vi "tdo -- V2.vi"() -> ()   [LabVIEW 2021]
uses:
  3-lorentzian-parameters.ctl
  filename-action.ctl
  nameformattingitem.ctl
  agregator -- action.ctl
  interpolation state - real.ctl
  tdo -- new/Data window.ctl
  <vilib>/Analysis/4window.llb/Hanning Window (DBL).vi
  <vilib>/Analysis/4window.llb/Blackman Window (DBL).vi
  linear interpolation - real -- V2.vi
  <vilib>/Analysis/4window.llb/AllCosWindow (DBL).vi
  <vilib>/Analysis/baseanly.llb/A x B.vi
  <vilib>/Analysis/baseanly.llb/Real A x B.vi
  Q -- check range -- i -- real.vi
  line -- complex.vi
  Q -- check range -- i -- integer.vi
  Q - not nan -- real.vi
  Q - not nan -- integer.vi
  <vilib>/measure/matone.llb/Extract Single Tone Information 1 Chan.vi
  <vilib>/Waveform/WDTOps.llb/WDT Number of Waveform Samples DBL.vi
  <vilib>/Utility/file.llb/Write Delimited Spreadsheet (string).vi
  <vilib>/Analysis/Matrix/Numeric/Conversions/Array To Matrix.vi
  <vilib>/Analysis/Matrix/Numeric/Conversions/Array To Matrix - RA2.vi
  <vilib>/Analysis/baseanly.llb/Inverse Matrix.vi
  <vilib>/Analysis/baseanly.llb/Real Inverse Matrix.vi
  <vilib>/Utility/file.llb/Write Delimited Spreadsheet (DBL).vi
  <vilib>/Analysis/NI_AALPro.lvlib
  <vilib>/measure/NI_MAPro.lvlib
  <vilib>/Analysis/NI_AAL_SigProc.lvlib
panel:
  in  "Tab Control":enum32{"Page 1", "Page 2", "Page 3", "Page 4"}(tab)
  in  "Tab Control 2":enum32{"Page 1", "Page 2"}(tab)
  in  "file pattern":string="p_c3*.tdms"
  in  "main folder":path=path "/Users/arkadyshekhter/Library/CloudStorage/Dropbox/shared_KimValBra/UTe2--Apr2024/april_2024"
  in  "readmathstring":bool=TRUE
  in  "selection :|\\":u16(ring)=31 caption="files" items=["p_c3_008_040924.tdms", "p_c3_003_041124.tdms", "p_c3_004_042224.tdms", "p_c3_005_042224.tdms", "p_c3_006_042224.tdms", "p_c3_007_042224.tdms", "p_c3_010_040924.tdms", "p_c3_008_042224.tdms", "p_c3_013_041024.tdms", "p_c3_004_041124.tdms", "p_c3_009_042224.tdms", "p_c3_006_041124.tdms", "p_c3_011_040924.tdms", "p_c3_010_042224.tdms", "p_c3_005_041124.tdms", "p_c3_012_041024.tdms", "p_c3_011_041024.tdms", "p_c3_002_041024.tdms", "p_c3_010_041024.tdms", "p_c3_009_041024.tdms", "p_c3_008_042524.tdms", "p_c3_007_041124.tdms", "p_c3_003_041024.tdms", "p_c3_007_042524.tdms", "p_c3_008_041124.tdms", "p_c3_006_042524.tdms", "p_c3_008_041024.tdms", "p_c3_005_042524.tdms", "p_c3_004_042524.tdms", "p_c3_007_041024.tdms", "p_c3_010_041124.tdms", "p_c3_003_041224.tdms", "p_c3_004_041224.tdms", "p_c3_005_041224.tdms", "p_c3_006_041224.tdms", "p_c3_007_041224.tdms", "p_c3_008_041224.tdms", "p_c3_009_041224.tdms", "p_c3_009_041124.tdms", "p_c3_011_041124.tdms", "p_c3_003_042524.tdms", "p_c3_004_041024.tdms", "p_c3_011_042224.tdms", "p_c3_013_042224.tdms", "p_c3_006_041024.tdms", "p_c3_002_041224.tdms", "p_c3_002_042524.tdms", "p_c3_004_042424.tdms", "p_c3_005_041024.tdms"]
  in  "file":path=path "/Users/arkadyshekhter/Library/CloudStorage/Dropbox/shared_KimValBra/UTe2--Apr2024/041224/p_c3_008_041224.tdms"
  out "T (K)":dbl=15.0 format="%#_3f"
  out "B (T)":dbl=60.0 format="%#_3f"
  out "θ (deg)":dbl=153.0 format="%#_3f"
  out "key":string="008_041224"
  in  "dothething! :' '":bool=TRUE
  in  "gamma window (sec)":dbl(slide)=0.00043000000000000004 scale=5e-05..0.001 scale format="%#_3p"
  out "E":cluster{dbl[], dbl[]}(graph)
  out "C":cluster{dbl[], dbl[]}(graph)
  out "A":cluster{dbl[], dbl[]}(graph)
  out "B":waveform(dbl)(graph)={"t0"=timestamp(-0.00999989999999995 s since 1904-01-01), "dt"=2e-05, "Y"=[]}
  out "Progress":dbl(slide)=1.004382311063316 scale=0.0..1.0
  in  "?":T1(tab)=enum."selectros"
  in  "Power spctr. threshold":dbl=0.0001 format="%.2p"
  in  "Freq. threshold":dbl=30000.0 format="%#_3p"
  in  "window width (s)":dbl=0.0003 format="%#_6p"
  in  "window step (s)":dbl=2e-05 format="%#_6p"
  in  "detection method":T2(ring)
  in  "fit width":i32=9 min=3
  in  "window type":enum16{"Hanning", "Box", "Blackman"}(ring)
  in  "what?":T3={"ignore set of !"=TRUE, "set (1T|2B)"=0, "ignore θ !"=TRUE, "ignore B !"=TRUE, "T (K)"=1.0, "ignore T !"=TRUE, "θ (∘)"=0.0, "B (T)"=0.0, "lookup"={"set of lookup"={0=1.0, 1=2.0}, "all set of"={0.0}, "T lookup"={0=0.12, 1=0.122, 2=0.14, 3=0.148, 4=0.15, 5=0.157, 6=0.16, 7=0.168, 8=0.17, 9=0.178, 10=0.179, 11=0.18, 12=0.19, 13=0.197, 14=0.2, 15=0.249, 16=0.25, 17=0.255, 18=0.26, 19=0.3, 20=0.307, 21=0.308, 22=0.31, 23=0.36, 24=0.42, 25=0.43, 26=0.438, 27=0.512, 28=0.52, 29=0.53, 30=0.61, 31=0.62, 32=0.63, 33=0.677, 34=0.81, 35=0.82, 36=0.83, 37=1.0, 38=1.1, 39=1.12, 40=1.13, 41=1.25, 42=1.28, 43=1.31, 44=1.39, 45=1.5, 46=1.52, 47=1.55, 48=1.6, 49=1.7, 50=1.8, 51=1.9, 52=2.1, 53=2.3, 54=3.0, 55=3.07, 56=3.1, 57=3.11, 58=5.5, 59=5.7, 60=5.75}, "θ lookup"={0=0.0, 1=30.0, 2=45.0, 3=60.0, 4=90.0}, "B lookup"={0=0.0, 1=1.0, 2=2.0, 3=4.0, 4=5.0, 5=6.0, 6=7.0, 7=8.0, 8=9.0, 9=10.0, 10=11.0, 11=12.0}, "all T's"={4.0, 10.0, 15.0, 17.0, 20.0, 25.0, 30.0}, "all θ's"={0.0, 15.0, 20.0, 25.0, 30.0, 40.0, 45.0, 50.0, 53.0, 55.0, 60.0, 65.0, 67.0, 75.0, 85.0, 90.0, 95.0, 105.0, 112.0, 120.0, 128.0, 135.0, 150.0, 151.0, 153.0, 155.0, 157.0, 160.0, 163.0, 165.0, 170.0, 180.0}, "all B's"={60.0}, "all sides"={4000.0, 8000.0}, "side lookup"={0=4000.0, 1=8000.0}}} {"B (T)" items=["0.000", "1.000", "2.000", "4.000", "5.000", "6.000", "7.000", "8.000", "9.000", "10.000", "11.000", "12.000"]; "θ (∘)" items=["0.000", "30.000", "45.000", "60.000", "90.000"]; "T (K)" items=["0.120", "0.122", "0.140", "0.148", "0.150", "0.157", "0.160", "0.168", "0.170", "0.178", "0.179", "0.180", "0.190", "0.197", "0.200", "0.249", "0.250", "0.255", "0.260", "0.300", "0.307", "0.308", "0.310", "0.360", "0.420", "0.430", "0.438", "0.512", "0.520", "0.530", "0.610", "0.620", "0.630", "0.677", "0.810", "0.820", "0.830", "1.000", "1.100", "1.120", "1.130", "1.250", "1.280", "1.310", "1.390", "1.500", "1.520", "1.550", "1.600", "1.700", "1.800", "1.900", "2.100", "2.300", "3.000", "3.070", "3.100", "3.110", "5.500", "5.700", "5.750"]; "set (1T|2B)" items=["1", "2"]}
  in  "X selector":T4=enum."θ (deg)"
  in  "ovewrite file?":bool=TRUE
  in  "add file suffix":string="_tdo_"
  in  "remove file prefix":string="p_c3_"
  out "first line":string[](array[string])=["<Not A Path>_time <Not A Path>_field <Not A Path>_freq <Not A Path>_amp <Not A Path>_gamma "]
  in  "field channel name":string="Field"
  in  "group name":string="p"
  in  "signal channel name":string="Vpick"
  in  "Field correction":dbl=1.0
  in  "Length for Bdot offset, s":dbl=0.009 format="%#_6p"
  out "D":waveform(dbl)(graph)={"t0"=timestamp(-0.00999989999999995 s since 1904-01-01), "dt"=2e-05, "Y"=[]}
  in  "Exit!":bool=TRUE
  in  "Low-pass filter":T5={"Clip IIR filter ramps, in 1/Tc units"=1.0, "Two-pass & flip"=TRUE, "IIR filter specifications"={"Topology"=enum."Off", "Type"=enum."Lowpass", "Order"=1, "Lower Fc"=1e-06, "Upper Fc"=0.0, "PB Ripple"=1.0, "SB Attenuation"=60.0}} {"IIR filter specifications"."PB Ripple" format="%0.2f"; "IIR filter specifications"."Lower Fc" format="%0.2p"; "IIR filter specifications"."SB Attenuation" format="%0.2f"; "IIR filter specifications"."Upper Fc" format="%0.2p"}
  in  "# of threads":i32=4
  out "Field profile":waveform(dbl)(graph)={"t0"=timestamp(-0.00999989999999995 s since 1904-01-01), "dt"=2e-05, "Y"=[]}
  out "all short filenames":map{string, string}(c390)={"002_041024"="p_c3_002_041024.tdms", "002_041224"="p_c3_002_041224.tdms", "002_042424"="p_c3_002_042424.tdms", "003_041024"="p_c3_003_041024.tdms", "003_041124"="p_c3_003_041124.tdms", "003_041224"="p_c3_003_041224.tdms", "003_042424"="p_c3_003_042424.tdms", "004_041024"="p_c3_004_041024.tdms", "004_041124"="p_c3_004_041124.tdms", "004_041224"="p_c3_004_041224.tdms", "004_042224"="p_c3_004_042224.tdms", "004_042424"="p_c3_004_042424.tdms", "005_041024"="p_c3_005_041024.tdms", "005_041124"="p_c3_005_041124.tdms", "005_041224"="p_c3_005_041224.tdms", "005_042224"="p_c3_005_042224.tdms", "006_041024"="p_c3_006_041024.tdms", "006_041124"="p_c3_006_041124.tdms", "006_041224"="p_c3_006_041224.tdms", "006_042224"="p_c3_006_042224.tdms", "007_041024"="p_c3_007_041024.tdms", "007_041124"="p_c3_007_041124.tdms", "007_041224"="p_c3_007_041224.tdms", "007_042224"="p_c3_007_042224.tdms", "008_040924"="p_c3_008_040924.tdms", "008_041024"="p_c3_008_041024.tdms", "008_041124"="p_c3_008_041124.tdms", "008_041224"="p_c3_008_041224.tdms", "008_042224"="p_c3_008_042224.tdms", "009_041024"="p_c3_009_041024.tdms", "009_041124"="p_c3_009_041124.tdms", "009_041224"="p_c3_009_041224.tdms", "009_042224"="p_c3_009_042224.tdms", "010_040924"="p_c3_010_040924.tdms", "010_041024"="p_c3_010_041024.tdms", "010_041124"="p_c3_010_041124.tdms", "010_042224"="p_c3_010_042224.tdms", "011_040924"="p_c3_011_040924.tdms", "011_041024"="p_c3_011_041024.tdms", "011_041124"="p_c3_011_041124.tdms", "011_042224"="p_c3_011_042224.tdms", "012_041024"="p_c3_012_041024.tdms", "013_041024"="p_c3_013_041024.tdms", "013_042224"="p_c3_013_042224.tdms"}
  out "temps&degs":map{string, map{T4, dbl}}(c390)={"002_041024"={enum."T (K)"=4.0, enum."B (T)"=60.0, enum."θ (deg)"=90.0, enum."plain"=23.0, enum."vproj"=0.0}, "002_041224"={enum."T (K)"=4.0, enum."B (T)"=60.0, enum."θ (deg)"=170.0, enum."plain"=23.0, enum."vproj"=-0.69}, "002_042424"={enum."T (K)"=4.0, enum."B (T)"=60.0, enum."θ (deg)"=170.0, enum."plain"=13.0, enum."vproj"=-0.692}, "003_041024"={enum."T (K)"=4.0, enum."B (T)"=60.0, enum."θ (deg)"=120.0, enum."plain"=23.0, enum."vproj"=-0.34}, "003_041124"={enum."T (K)"=4.0, enum."B (T)"=60.0, enum."θ (deg)"=15.0, enum."plain"=23.0, enum."vproj"=0.673}, "003_041224"={enum."T (K)"=4.0, enum."B (T)"=60.0, enum."θ (deg)"=153.0, enum."plain"=23.0, enum."vproj"=-0.625}, "003_042424"={enum."T (K)"=4.0, enum."B (T)"=60.0, enum."θ (deg)"=160.0, enum."plain"=13.0, enum."vproj"=-0.662}, "004_041024"={enum."T (K)"=4.0, enum."B (T)"=60.0, enum."θ (deg)"=160.0, enum."plain"=23.0, enum."vproj"=-0.663}, "004_041124"={enum."T (K)"=4.0, enum."B (T)"=60.0, enum."θ (deg)"=50.0, enum."plain"=23.0, enum."vproj"=0.442}, "004_041224"={enum."T (K)"=10.0, enum."B (T)"=60.0, enum."θ (deg)"=153.0, enum."plain"=23.0, enum."vproj"=-0.625}, "004_042224"={enum."T (K)"=4.0, enum."B (T)"=60.0, enum."θ (deg)"=15.0, enum."plain"=23.0, enum."vproj"=0.67}, "004_042424"={enum."T (K)"=4.0, enum."B (T)"=60.0, enum."θ (deg)"=180.0, enum."plain"=13.0, enum."vproj"=-0.702}, "005_041024"={enum."T (K)"=4.0, enum."B (T)"=60.0, enum."θ (deg)"=180.0, enum."plain"=23.0, enum."vproj"=-0.699}, "005_041124"={enum."T (K)"=4.0, enum."B (T)"=60.0, enum."θ (deg)"=67.0, enum."plain"=23.0, enum."vproj"=0.269}, "005_041224"={enum."T (K)"=20.0, enum."B (T)"=60.0, enum."θ (deg)"=153.0, enum."plain"=23.0, enum."vproj"=-0.625}, "005_042224"={enum."T (K)"=4.0, enum."B (T)"=60.0, enum."θ (deg)"=20.0, enum."plain"=23.0, enum."vproj"=0.651}, "006_041024"={enum."T (K)"=4.0, enum."B (T)"=60.0, enum."θ (deg)"=165.0, enum."plain"=23.0, enum."vproj"=-0.677}, "006_041124"={enum."T (K)"=4.0, enum."B (T)"=60.0, enum."θ (deg)"=55.0, enum."plain"=23.0, enum."vproj"=0.397}, "006_041224"={enum."T (K)"=30.0, enum."B (T)"=60.0, enum."θ (deg)"=153.0, enum."plain"=23.0, enum."vproj"=-0.625}, "006_042224"={enum."T (K)"=4.0, enum."B (T)"=60.0, enum."θ (deg)"=25.0, enum."plain"=23.0, enum."vproj"=0.628}, "007_041024"={enum."T (K)"=4.0, enum."B (T)"=60.0, enum."θ (deg)"=150.0, enum."plain"=23.0, enum."vproj"=-0.603}, "007_041124"={enum."T (K)"=4.0, enum."B (T)"=60.0, enum."θ (deg)"=112.0, enum."plain"=23.0, enum."vproj"=-0.26}, "007_041224"={enum."T (K)"=25.0, enum."B (T)"=60.0, enum."θ (deg)"=153.0, enum."plain"=23.0, enum."vproj"=-0.625}, "007_042224"={enum."T (K)"=4.0, enum."B (T)"=60.0, enum."θ (deg)"=30.0, enum."plain"=23.0, enum."vproj"=0.603}, "008_040924"={enum."T (K)"=4.0, enum."B (T)"=60.0, enum."θ (deg)"=0.0, enum."plain"=23.0, enum."vproj"=0.69}, "008_041024"={enum."T (K)"=4.0, enum."B (T)"=60.0, enum."θ (deg)"=135.0, enum."plain"=23.0, enum."vproj"=-0.496}, "008_041124"={enum."T (K)"=4.0, enum."B (T)"=60.0, enum."θ (deg)"=128.0, enum."plain"=23.0, enum."vproj"=-0.432}, "008_041224"={enum."T (K)"=15.0, enum."B (T)"=60.0, enum."θ (deg)"=153.0, enum."plain"=23.0, enum."vproj"=-0.625}, "008_042224"={enum."T (K)"=4.0, enum."B (T)"=60.0, enum."θ (deg)"=40.0, enum."plain"=23.0, enum."vproj"=0.533}, "009_041024"={enum."T (K)"=4.0, enum."B (T)"=60.0, enum."θ (deg)"=105.0, enum."plain"=23.0, enum."vproj"=-0.178}, "009_041124"={enum."T (K)"=4.0, enum."B (T)"=60.0, enum."θ (deg)"=155.0, enum."plain"=23.0, enum."vproj"=-0.634}, "009_041224"={enum."T (K)"=17.0, enum."B (T)"=60.0, enum."θ (deg)"=153.0, enum."plain"=23.0, enum."vproj"=-0.625}, "009_042224"={enum."T (K)"=4.0, enum."B (T)"=60.0, enum."θ (deg)"=53.0, enum."plain"=23.0, enum."vproj"=0.415}, "010_040924"={enum."T (K)"=4.0, enum."B (T)"=60.0, enum."θ (deg)"=30.0, enum."plain"=23.0, enum."vproj"=0.6}, "010_041024"={enum."T (K)"=4.0, enum."B (T)"=60.0, enum."θ (deg)"=95.0, enum."plain"=23.0, enum."vproj"=-0.057}, "010_041124"={enum."T (K)"=4.0, enum."B (T)"=60.0, enum."θ (deg)"=151.0, enum."plain"=23.0, enum."vproj"=-0.615}, "010_042224"={enum."T (K)"=4.0, enum."B (T)"=60.0, enum."θ (deg)"=65.0, enum."plain"=23.0, enum."vproj"=0.288}, "011_040924"={enum."T (K)"=4.0, enum."B (T)"=60.0, enum."θ (deg)"=60.0, enum."plain"=23.0, enum."vproj"=0.348}, "011_041024"={enum."T (K)"=4.0, enum."B (T)"=60.0, enum."θ (deg)"=85.0, enum."plain"=23.0, enum."vproj"=0.065}, "011_041124"={enum."T (K)"=4.0, enum."B (T)"=60.0, enum."θ (deg)"=157.0, enum."plain"=23.0, enum."vproj"=-0.648}, "011_042224"={enum."T (K)"=4.0, enum."B (T)"=60.0, enum."θ (deg)"=160.0, enum."plain"=23.0, enum."vproj"=-0.661}, "012_041024"={enum."T (K)"=4.0, enum."B (T)"=60.0, enum."θ (deg)"=75.0, enum."plain"=23.0, enum."vproj"=0.183}, "013_041024"={enum."T (K)"=4.0, enum."B (T)"=60.0, enum."θ (deg)"=45.0, enum."plain"=23.0, enum."vproj"=0.494}, "013_042224"={enum."T (K)"=4.0, enum."B (T)"=60.0, enum."θ (deg)"=163.0, enum."plain"=23.0, enum."vproj"=-0.674}}
  out "mathematica thing":map{string, map{T4, dbl}}(c390)={"002_041024"={enum."T (K)"=4.0, enum."B (T)"=60.0, enum."θ (deg)"=90.0, enum."plain"=23.0, enum."vproj"=0.0}, "002_041224"={enum."T (K)"=4.0, enum."B (T)"=60.0, enum."θ (deg)"=170.0, enum."plain"=23.0, enum."vproj"=-0.69}, "002_042424"={enum."T (K)"=4.0, enum."B (T)"=60.0, enum."θ (deg)"=170.0, enum."plain"=13.0, enum."vproj"=-0.692}, "003_041024"={enum."T (K)"=4.0, enum."B (T)"=60.0, enum."θ (deg)"=120.0, enum."plain"=23.0, enum."vproj"=-0.34}, "003_041124"={enum."T (K)"=4.0, enum."B (T)"=60.0, enum."θ (deg)"=15.0, enum."plain"=23.0, enum."vproj"=0.673}, "003_041224"={enum."T (K)"=4.0, enum."B (T)"=60.0, enum."θ (deg)"=153.0, enum."plain"=23.0, enum."vproj"=-0.625}, "003_042424"={enum."T (K)"=4.0, enum."B (T)"=60.0, enum."θ (deg)"=160.0, enum."plain"=13.0, enum."vproj"=-0.662}, "004_041024"={enum."T (K)"=4.0, enum."B (T)"=60.0, enum."θ (deg)"=160.0, enum."plain"=23.0, enum."vproj"=-0.663}, "004_041124"={enum."T (K)"=4.0, enum."B (T)"=60.0, enum."θ (deg)"=50.0, enum."plain"=23.0, enum."vproj"=0.442}, "004_041224"={enum."T (K)"=10.0, enum."B (T)"=60.0, enum."θ (deg)"=153.0, enum."plain"=23.0, enum."vproj"=-0.625}, "004_042224"={enum."T (K)"=4.0, enum."B (T)"=60.0, enum."θ (deg)"=15.0, enum."plain"=23.0, enum."vproj"=0.67}, "004_042424"={enum."T (K)"=4.0, enum."B (T)"=60.0, enum."θ (deg)"=180.0, enum."plain"=13.0, enum."vproj"=-0.702}, "005_041024"={enum."T (K)"=4.0, enum."B (T)"=60.0, enum."θ (deg)"=180.0, enum."plain"=23.0, enum."vproj"=-0.699}, "005_041124"={enum."T (K)"=4.0, enum."B (T)"=60.0, enum."θ (deg)"=67.0, enum."plain"=23.0, enum."vproj"=0.269}, "005_041224"={enum."T (K)"=20.0, enum."B (T)"=60.0, enum."θ (deg)"=153.0, enum."plain"=23.0, enum."vproj"=-0.625}, "005_042224"={enum."T (K)"=4.0, enum."B (T)"=60.0, enum."θ (deg)"=20.0, enum."plain"=23.0, enum."vproj"=0.651}, "006_041024"={enum."T (K)"=4.0, enum."B (T)"=60.0, enum."θ (deg)"=165.0, enum."plain"=23.0, enum."vproj"=-0.677}, "006_041124"={enum."T (K)"=4.0, enum."B (T)"=60.0, enum."θ (deg)"=55.0, enum."plain"=23.0, enum."vproj"=0.397}, "006_041224"={enum."T (K)"=30.0, enum."B (T)"=60.0, enum."θ (deg)"=153.0, enum."plain"=23.0, enum."vproj"=-0.625}, "006_042224"={enum."T (K)"=4.0, enum."B (T)"=60.0, enum."θ (deg)"=25.0, enum."plain"=23.0, enum."vproj"=0.628}, "007_041024"={enum."T (K)"=4.0, enum."B (T)"=60.0, enum."θ (deg)"=150.0, enum."plain"=23.0, enum."vproj"=-0.603}, "007_041124"={enum."T (K)"=4.0, enum."B (T)"=60.0, enum."θ (deg)"=112.0, enum."plain"=23.0, enum."vproj"=-0.26}, "007_041224"={enum."T (K)"=25.0, enum."B (T)"=60.0, enum."θ (deg)"=153.0, enum."plain"=23.0, enum."vproj"=-0.625}, "007_042224"={enum."T (K)"=4.0, enum."B (T)"=60.0, enum."θ (deg)"=30.0, enum."plain"=23.0, enum."vproj"=0.603}, "008_040924"={enum."T (K)"=4.0, enum."B (T)"=60.0, enum."θ (deg)"=0.0, enum."plain"=23.0, enum."vproj"=0.69}, "008_041024"={enum."T (K)"=4.0, enum."B (T)"=60.0, enum."θ (deg)"=135.0, enum."plain"=23.0, enum."vproj"=-0.496}, "008_041124"={enum."T (K)"=4.0, enum."B (T)"=60.0, enum."θ (deg)"=128.0, enum."plain"=23.0, enum."vproj"=-0.432}, "008_041224"={enum."T (K)"=15.0, enum."B (T)"=60.0, enum."θ (deg)"=153.0, enum."plain"=23.0, enum."vproj"=-0.625}, "008_042224"={enum."T (K)"=4.0, enum."B (T)"=60.0, enum."θ (deg)"=40.0, enum."plain"=23.0, enum."vproj"=0.533}, "009_041024"={enum."T (K)"=4.0, enum."B (T)"=60.0, enum."θ (deg)"=105.0, enum."plain"=23.0, enum."vproj"=-0.178}, "009_041124"={enum."T (K)"=4.0, enum."B (T)"=60.0, enum."θ (deg)"=155.0, enum."plain"=23.0, enum."vproj"=-0.634}, "009_041224"={enum."T (K)"=17.0, enum."B (T)"=60.0, enum."θ (deg)"=153.0, enum."plain"=23.0, enum."vproj"=-0.625}, "009_042224"={enum."T (K)"=4.0, enum."B (T)"=60.0, enum."θ (deg)"=53.0, enum."plain"=23.0, enum."vproj"=0.415}, "010_040924"={enum."T (K)"=4.0, enum."B (T)"=60.0, enum."θ (deg)"=30.0, enum."plain"=23.0, enum."vproj"=0.6}, "010_041024"={enum."T (K)"=4.0, enum."B (T)"=60.0, enum."θ (deg)"=95.0, enum."plain"=23.0, enum."vproj"=-0.057}, "010_041124"={enum."T (K)"=4.0, enum."B (T)"=60.0, enum."θ (deg)"=151.0, enum."plain"=23.0, enum."vproj"=-0.615}, "010_042224"={enum."T (K)"=4.0, enum."B (T)"=60.0, enum."θ (deg)"=65.0, enum."plain"=23.0, enum."vproj"=0.288}, "011_040924"={enum."T (K)"=4.0, enum."B (T)"=60.0, enum."θ (deg)"=60.0, enum."plain"=23.0, enum."vproj"=0.348}, "011_041024"={enum."T (K)"=4.0, enum."B (T)"=60.0, enum."θ (deg)"=85.0, enum."plain"=23.0, enum."vproj"=0.065}, "011_041124"={enum."T (K)"=4.0, enum."B (T)"=60.0, enum."θ (deg)"=157.0, enum."plain"=23.0, enum."vproj"=-0.648}, "011_042224"={enum."T (K)"=4.0, enum."B (T)"=60.0, enum."θ (deg)"=160.0, enum."plain"=23.0, enum."vproj"=-0.661}, "012_041024"={enum."T (K)"=4.0, enum."B (T)"=60.0, enum."θ (deg)"=75.0, enum."plain"=23.0, enum."vproj"=0.183}, "013_041024"={enum."T (K)"=4.0, enum."B (T)"=60.0, enum."θ (deg)"=45.0, enum."plain"=23.0, enum."vproj"=0.494}, "013_042224"={enum."T (K)"=4.0, enum."B (T)"=60.0, enum."θ (deg)"=163.0, enum."plain"=23.0, enum."vproj"=-0.674}}
  out "all full filenames":map{string, path}(c390)={"002_041024"=path "/Users/arkadyshekhter/Library/CloudStorage/Dropbox/shared_KimValBra/UTe2--Apr2024/041024/p_c3_002_041024.tdms", "002_041224"=path "/Users/arkadyshekhter/Library/CloudStorage/Dropbox/shared_KimValBra/UTe2--Apr2024/041224/p_c3_002_041224.tdms", "002_042424"=path "/Users/arkadyshekhter/Library/CloudStorage/Dropbox/shared_KimValBra/UTe2--Apr2024/042424/p_c3_002_042424.tdms", "003_041024"=path "/Users/arkadyshekhter/Library/CloudStorage/Dropbox/shared_KimValBra/UTe2--Apr2024/041024/p_c3_003_041024.tdms", "003_041124"=path "/Users/arkadyshekhter/Library/CloudStorage/Dropbox/shared_KimValBra/UTe2--Apr2024/041124/p_c3_003_041124.tdms", "003_041224"=path "/Users/arkadyshekhter/Library/CloudStorage/Dropbox/shared_KimValBra/UTe2--Apr2024/041224/p_c3_003_041224.tdms", "003_042424"=path "/Users/arkadyshekhter/Library/CloudStorage/Dropbox/shared_KimValBra/UTe2--Apr2024/042424/p_c3_003_042424.tdms", "004_041024"=path "/Users/arkadyshekhter/Library/CloudStorage/Dropbox/shared_KimValBra/UTe2--Apr2024/041024/p_c3_004_041024.tdms", "004_041124"=path "/Users/arkadyshekhter/Library/CloudStorage/Dropbox/shared_KimValBra/UTe2--Apr2024/041124/p_c3_004_041124.tdms", "004_041224"=path "/Users/arkadyshekhter/Library/CloudStorage/Dropbox/shared_KimValBra/UTe2--Apr2024/041224/p_c3_004_041224.tdms", "004_042224"=path "/Users/arkadyshekhter/Library/CloudStorage/Dropbox/shared_KimValBra/UTe2--Apr2024/042224/p_c3_004_042224.tdms", "004_042424"=path "/Users/arkadyshekhter/Library/CloudStorage/Dropbox/shared_KimValBra/UTe2--Apr2024/042424/p_c3_004_042424.tdms", "005_041024"=path "/Users/arkadyshekhter/Library/CloudStorage/Dropbox/shared_KimValBra/UTe2--Apr2024/041024/p_c3_005_041024.tdms", "005_041124"=path "/Users/arkadyshekhter/Library/CloudStorage/Dropbox/shared_KimValBra/UTe2--Apr2024/041124/p_c3_005_041124.tdms", "005_041224"=path "/Users/arkadyshekhter/Library/CloudStorage/Dropbox/shared_KimValBra/UTe2--Apr2024/041224/p_c3_005_041224.tdms", "005_042224"=path "/Users/arkadyshekhter/Library/CloudStorage/Dropbox/shared_KimValBra/UTe2--Apr2024/042224/p_c3_005_042224.tdms", "006_041024"=path "/Users/arkadyshekhter/Library/CloudStorage/Dropbox/shared_KimValBra/UTe2--Apr2024/041024/p_c3_006_041024.tdms", "006_041124"=path "/Users/arkadyshekhter/Library/CloudStorage/Dropbox/shared_KimValBra/UTe2--Apr2024/041124/p_c3_006_041124.tdms", "006_041224"=path "/Users/arkadyshekhter/Library/CloudStorage/Dropbox/shared_KimValBra/UTe2--Apr2024/041224/p_c3_006_041224.tdms", "006_042224"=path "/Users/arkadyshekhter/Library/CloudStorage/Dropbox/shared_KimValBra/UTe2--Apr2024/042224/p_c3_006_042224.tdms", "007_041024"=path "/Users/arkadyshekhter/Library/CloudStorage/Dropbox/shared_KimValBra/UTe2--Apr2024/041024/p_c3_007_041024.tdms", "007_041124"=path "/Users/arkadyshekhter/Library/CloudStorage/Dropbox/shared_KimValBra/UTe2--Apr2024/041124/p_c3_007_041124.tdms", "007_041224"=path "/Users/arkadyshekhter/Library/CloudStorage/Dropbox/shared_KimValBra/UTe2--Apr2024/041224/p_c3_007_041224.tdms", "007_042224"=path "/Users/arkadyshekhter/Library/CloudStorage/Dropbox/shared_KimValBra/UTe2--Apr2024/042224/p_c3_007_042224.tdms", "008_040924"=path "/Users/arkadyshekhter/Library/CloudStorage/Dropbox/shared_KimValBra/UTe2--Apr2024/040924/p_c3_008_040924.tdms", "008_041024"=path "/Users/arkadyshekhter/Library/CloudStorage/Dropbox/shared_KimValBra/UTe2--Apr2024/041024/p_c3_008_041024.tdms", "008_041124"=path "/Users/arkadyshekhter/Library/CloudStorage/Dropbox/shared_KimValBra/UTe2--Apr2024/041124/p_c3_008_041124.tdms", "008_041224"=path "/Users/arkadyshekhter/Library/CloudStorage/Dropbox/shared_KimValBra/UTe2--Apr2024/041224/p_c3_008_041224.tdms", "008_042224"=path "/Users/arkadyshekhter/Library/CloudStorage/Dropbox/shared_KimValBra/UTe2--Apr2024/042224/p_c3_008_042224.tdms", "009_041024"=path "/Users/arkadyshekhter/Library/CloudStorage/Dropbox/shared_KimValBra/UTe2--Apr2024/041024/p_c3_009_041024.tdms", "009_041124"=path "/Users/arkadyshekhter/Library/CloudStorage/Dropbox/shared_KimValBra/UTe2--Apr2024/041124/p_c3_009_041124.tdms", "009_041224"=path "/Users/arkadyshekhter/Library/CloudStorage/Dropbox/shared_KimValBra/UTe2--Apr2024/041224/p_c3_009_041224.tdms", "009_042224"=path "/Users/arkadyshekhter/Library/CloudStorage/Dropbox/shared_KimValBra/UTe2--Apr2024/042224/p_c3_009_042224.tdms", "010_040924"=path "/Users/arkadyshekhter/Library/CloudStorage/Dropbox/shared_KimValBra/UTe2--Apr2024/040924/p_c3_010_040924.tdms", "010_041024"=path "/Users/arkadyshekhter/Library/CloudStorage/Dropbox/shared_KimValBra/UTe2--Apr2024/041024/p_c3_010_041024.tdms", "010_041124"=path "/Users/arkadyshekhter/Library/CloudStorage/Dropbox/shared_KimValBra/UTe2--Apr2024/041124/p_c3_010_041124.tdms", "010_042224"=path "/Users/arkadyshekhter/Library/CloudStorage/Dropbox/shared_KimValBra/UTe2--Apr2024/042224/p_c3_010_042224.tdms", "011_040924"=path "/Users/arkadyshekhter/Library/CloudStorage/Dropbox/shared_KimValBra/UTe2--Apr2024/040924/p_c3_011_040924.tdms", "011_041024"=path "/Users/arkadyshekhter/Library/CloudStorage/Dropbox/shared_KimValBra/UTe2--Apr2024/041024/p_c3_011_041024.tdms", "011_041124"=path "/Users/arkadyshekhter/Library/CloudStorage/Dropbox/shared_KimValBra/UTe2--Apr2024/041124/p_c3_011_041124.tdms", "011_042224"=path "/Users/arkadyshekhter/Library/CloudStorage/Dropbox/shared_KimValBra/UTe2--Apr2024/042224/p_c3_011_042224.tdms", "012_041024"=path "/Users/arkadyshekhter/Library/CloudStorage/Dropbox/shared_KimValBra/UTe2--Apr2024/041024/p_c3_012_041024.tdms", "013_041024"=path "/Users/arkadyshekhter/Library/CloudStorage/Dropbox/shared_KimValBra/UTe2--Apr2024/041024/p_c3_013_041024.tdms", "013_042224"=path "/Users/arkadyshekhter/Library/CloudStorage/Dropbox/shared_KimValBra/UTe2--Apr2024/042224/p_c3_013_042224.tdms"}
  in  "string IN":string="\"002_042424\" ->   <|  \n\"T\"->  4.0  , \n\"θ\"-> 170 , \n\"vproj\"  -> -0.692,\n\"B\" -> 60 ,\n\"plain\" -> 13\n  |>   , \n  \n\"003_042424\" ->   <|  \n\"T\"->  4.0  , \n\"θ\"-> 160 , \n\"vproj\"  -> -0.662,\n\"B\" -> 60 , \n\"plain\" -> 13\n  |>   , \n  \n\"004_042424\" ->   <|  \n\"T\"->  4.0  , \n\"θ\"-> 150 , \n\"vproj\"  -> -0.608,\n\"B\" -> 60 , \n\"plain\" -> 13\n  |>   , \n  \n\"004_042424\" ->   <|  \n\"T\"->  4.0  , \n\"θ\"-> 180 , \n\"vproj\"  -> -0.702,\n\"B\" -> 60 , \n\"plain\" -> 13\n  |>   , \n  \n\n\n\"008_040924\" ->   <|  \n\"T\"->  4.0  , \n\"θ\"-> 0 , \n\"vproj\"  -> 0.690,\n\"B\" -> 60 ,\n\"plain\" -> 23\n  |>   , \n  \n    \n\"010_040924\" ->   <|  \n\"T\"->  4.0  , \n\"θ\"-> 30  , \n\"vproj\"  -> 0.600,\n\"B\" -> 60 ,\n\"plain\" -> 23\n  |>   , \n  \n\"011_040924\" ->   <|  \n\"T\"->  4.0  , \n\"θ\"-> 60  , \n\"vproj\"  -> 0.348,\n\"B\" -> 60 ,\n\"plain\" -> 23\n  |>   ,   \n  \n  \n\"002_041024\" ->   <|  \n\"T\"->  4.0  , \n\"θ\"-> 90  , \n\"vproj\"  -> 0.00,\n\"B\" -> 60 ,\n\"plain\" -> 23\n  |>   ,\n   \n    \n\"003_041024\" ->   <|  \n\"T\"->  4.0  , \n\"θ\"-> 120  , \n\"vproj\"  -> -0.340,\n\"B\" -> 60 ,\n\"plain\" -> 23\n  |>   ,\n\n\"004_041024\" ->   <|  \n\"T\"->  4.0  , \n\"θ\"-> 160  , \n\"vproj\"  -> -0.663,\n\"B\" -> 60 ,\n\"plain\" -> 23\n  |>   , \n  \n\"005_041024\" ->   <|  \n\"T\"->  4.0  , \n\"θ\"-> 180  , \n\"vproj\"  -> -0.699,\n\"B\" -> 60 ,\n\"plain\" -> 23\n  |>   , \n  \n\"006_041024\" ->   <|  \n\"T\"->  4.0  , \n\"θ\"-> 165  , \n\"vproj\"  -> -0.677,\n\"B\" -> 60 ,\n\"plain\" -> 23\n  |>   ,\n  \n\"007_041024\" ->   <|  \n\"T\"->  4.0  , \n\"θ\"-> 150  , \n\"vproj\"  -> -0.603,\n\"B\" -> 60 ,\n\"plain\" -> 23\n  |>   ,\n  \n\"008_041024\" ->   <|  \n\"T\"->  4.0  , \n\"θ\"-> 135  , \n\"vproj\"  -> -0.496,\n\"B\" -> 60 ,\n\"plain\" -> 23\n  |>   ,\n  \n\"009_041024\" ->   <|  \n\"T\"->  4.0  , \n\"θ\"-> 105  , \n\"vproj\"  -> -0.178,\n\"B\" -> 60 ,\n\"plain\" -> 23\n  |>   ,\n  \n\"010_041024\" ->   <|  \n\"T\"->  4.0  , \n\"θ\"-> 95  , \n\"vproj\"  -> -0.057,\n\"B\" -> 60 ,\n\"plain\" -> 23\n  |>   ,\n  \n\"011_041024\" ->   <|  \n\"T\"->  4.0  , \n\"θ\"-> 85  , \n\"vproj\"  -> +0.065,\n\"B\" -> 60 ,\n\"plain\" -> 23\n  |>   ,\n  \n\"012_041024\" ->   <|  \n\"T\"->  4.0  , \n\"θ\"-> 75  , \n\"vproj\"  -> +0.183,\n\"B\" -> 60 ,\n\"plain\" -> 23\n  |>   , \n  \n\"013_041024\" ->   <|  \n\"T\"->  4.0  , \n\"θ\"-> 45  , \n\"vproj\"  -> +0.494,\n\"B\" -> 60 ,\n\"plain\" -> 23\n  |>   , \n  \n\"003_041124\" ->   <|  \n\"T\"->  4.0  , \n\"θ\"-> 15  , \n\"vproj\"  -> +0.673,\n\"B\" -> 60 ,\n\"plain\" -> 23\n  |>   ,  \n  \n\"004_041124\" ->   <|  \n\"T\"->  4.0  , \n\"θ\"-> 50  , \n\"vproj\"  -> +0.442,\n\"B\" -> 60 ,\n\"plain\" -> 23\n  |>   ,\n  \n\"005_041124\" ->   <|  \n\"T\"->  4.0  , \n\"θ\"-> 67  , \n\"vproj\"  -> +0.269,\n\"B\" -> 60 ,\n\"plain\" -> 23\n  |>   ,\n  \n\"006_041124\" ->   <|  \n\"T\"->  4.0  , \n\"θ\"-> 55  , \n\"vproj\"  -> +0.397,\n\"B\" -> 60 ,\n\"plain\" -> 23\n  |>   ,   \n  \n\"007_041124\" ->   <|  \n\"T\"->  4.0  , \n\"θ\"-> 112  , \n\"vproj\"  -> -0.260,\n\"B\" -> 60 ,\n\"plain\" -> 23\n  |>   ,  \n  \n\"008_041124\" ->   <|  \n\"T\"->  4.0  , \n\"θ\"-> 128  , \n\"vproj\"  -> -0.432,\n\"B\" -> 60 ,\n\"plain\" -> 23\n  |>   , \n  \n\"009_041124\" ->   <|  \n\"T\"->  4.0  , \n\"θ\"-> 155  , \n\"vproj\"  -> -0.634,\n\"B\" -> 60 ,\n\"plain\" -> 23\n  |>   , \n  \n\"010_041124\" ->   <|  \n\"T\"->  4.0  , \n\"θ\"-> 151  , \n\"vproj\"  -> -0.615,\n\"B\" -> 60 ,\n\"plain\" -> 23\n  |>   ,   \n  \n\"011_041124\" ->   <|  \n\"T\"->  4.0  , \n\"θ\"-> 157  , \n\"vproj\"  -> -0.648,\n\"B\" -> 60 ,\n\"plain\" -> 23\n  |>   ,  \n  \n  \n\"002_041224\" ->   <|  \n\"T\"->  4.0  , \n\"θ\"-> 170  , \n\"vproj\"  -> -0.690,\n\"B\" -> 60 ,\n\"plain\" -> 23\n  |>   ,\n  \n\"003_041224\" ->   <|  \n\"T\"->  4.0  , \n\"θ\"-> 153  , \n\"vproj\"  -> -0.625,\n\"B\" -> 60 ,\n\"plain\" -> 23\n  |>   , \n  \n  \n\"004_041224\" ->   <|  \n\"T\"->  10.0  , \n\"θ\"-> 153  , \n\"vproj\"  -> -0.625,\n\"B\" -> 60 ,\n\"plain\" -> 23\n  |>   ,\n  \n  \n\"005_041224\" ->   <|  \n\"T\"->  20.0  , \n\"θ\"-> 153  , \n\"vproj\"  -> -0.625,\n\"B\" -> 60 ,\n\"plain\" -> 23\n  |>   , \n  \n\"006_041224\" ->   <|  \n\"T\"->  30.0  , \n\"θ\"-> 153  , \n\"vproj\"  -> -0.625,\n\"B\" -> 60 ,\n\"plain\" -> 23\n  |>   ,\n  \n  \n\"007_041224\" ->   <|  \n\"T\"->  25.0  , \n\"θ\"-> 153  , \n\"vproj\"  -> -0.625,\n\"B\" -> 60 ,\n\"plain\" -> 23\n  |>   , \n  \n  \n\"008_041224\" ->   <|  \n\"T\"->  15.0  , \n\"θ\"-> 153  , \n\"vproj\"  -> -0.625,\n\"B\" -> 60 ,\n\"plain\" -> 23\n  |>   , \n  \n  \n\"009_041224\" ->   <|  \n\"T\"->  17.0  , \n\"θ\"-> 153  , \n\"vproj\"  -> -0.625,\n\"B\" -> 60 ,\n\"plain\" -> 23\n  |>   , \n  \n  \n  \n  \n\"004_042224\" ->   <|  \n\"T\"->  4.0  , \n\"θ\"-> 15  , \n\"vproj\"  -> +0.670,\n\"B\" -> 60 ,\n\"plain\" -> 23\n  |>   ,   \n  \n  \n\"005_042224\" ->   <|  \n\"T\"->  4.0  , \n\"θ\"-> 20  , \n\"vproj\"  -> +0.651,\n\"B\" -> 60 ,\n\"plain\" -> 23\n  |>   ,\n  \n\"006_042224\" ->   <|  \n\"T\"->  4.0  , \n\"θ\"-> 25  , \n\"vproj\"  -> +0.628,\n\"B\" -> 60 ,\n\"plain\" -> 23\n  |>   ,\n  \n  \n\"007_042224\" ->   <|  \n\"T\"->  4.0  , \n\"θ\"-> 30  , \n\"vproj\"  -> +0.603,\n\"B\" -> 60 ,\n\"plain\" -> 23\n  |>   , \n  \n\"008_042224\" ->   <|  \n\"T\"->  4.0  , \n\"θ\"-> 40  , \n\"vproj\"  -> +0.533,\n\"B\" -> 60 ,\n\"plain\" -> 23\n  |>   ,\n  \n  \n  \n\"009_042224\" ->   <|  \n\"T\"->  4.0  , \n\"θ\"-> 53  , \n\"vproj\"  -> +0.415,\n\"B\" -> 60 ,\n\"plain\" -> 23\n  |>   , \n  \n  \n\"010_042224\" ->   <|  \n\"T\"->  4.0  , \n\"θ\"-> 65  , \n\"vproj\"  -> +0.288,\n\"B\" -> 60 ,\n\"plain\" -> 23\n  |>   ,   \n  \n  \n\"011_042224\" ->   <|  \n\"T\"->  4.0  , \n\"θ\"-> 160  , \n\"vproj\"  -> -0.661,\n\"B\" -> 60 ,\n\"plain\" -> 23\n  |>   ,  \n  \n  \n\"013_042224\" ->   <|  \n\"T\"->  4.0  , \n\"θ\"-> 163  , \n\"vproj\"  -> -0.674,\n\"B\" -> 60 ,\n\"plain\" -> 23\n  |>   ,                                                               \n                                              \n                                   "
  out "data file parameters map":map{T4, T6}(c390)={enum."T (K)"=enum."get T", enum."B (T)"=enum."get B", enum."θ (deg)"=enum."get deg", enum."plain"=enum."getplain", enum."vproj"=enum."getvproj"}
  out "state of all selectors":map{T4, map{bool, dbl}}(c390)={enum."T (K)"={TRUE=0.122}, enum."B (T)"={TRUE=0.0}, enum."θ (deg)"={TRUE=0.0}, enum."set of (B|T)"={TRUE=1.0}}
  out "state of all selectors string":string="__0.000au__0.000V_"
  out "new selector names":map{T4, map{T7, string}}(c390)={enum."ζ"={enum."name"="ζ", enum."nameL"="zeta", enum."units"="sec", enum."prec"="%_4p"}, enum."τ1"={enum."name"="τ1", enum."nameL"="tau1", enum."units"="sec", enum."prec"="%_4p"}, enum."τS"={enum."name"="τS", enum."nameL"="tauS", enum."units"="sec", enum."prec"="%_4p"}, enum."τN"={enum."name"="τN", enum."nameL"="tauN", enum."units"="sec", enum."prec"="%_4p"}, enum."τC"={enum."name"="τC", enum."nameL"="tauC", enum."units"="sec", enum."prec"="%_4p"}, enum."κ0"={enum."name"="κ0", enum."nameL"="kappa0", enum."units"="WperK", enum."prec"="%_5p"}, enum."T (K)"={enum."name"="T", enum."nameL"="T", enum."units"="K", enum."prec"="%_4p"}, enum."B (T)"={enum."name"="B", enum."nameL"="B", enum."units"="T", enum."prec"="%_2p"}, enum."θ (deg)"={enum."name"="θ", enum."nameL"="theta", enum."units"="deg", enum."prec"="%_2p"}, enum."side (S|R)"={enum."name"="side", enum."nameL"="side", enum."units"="side", enum."prec"="%d"}, enum."Re(offset)"={enum."name"="Reoffset", enum."nameL"="Reoffset", enum."units"="au", enum."prec"="%_4p"}, enum."Im(offset)"={enum."name"="Imoffset", enum."nameL"="Imoffset", enum."units"="au", enum."prec"="%_4p"}, enum."στ1"={enum."name"="στ1", enum."nameL"="sigmatau1", enum."units"="sec", enum."prec"="%_4p"}, enum."στS"={enum."name"="στS", enum."nameL"="sigmatauS", enum."units"="sec", enum."prec"="%_4p"}, enum."στN"={enum."name"="στN", enum."nameL"="sigmatauN", enum."units"="sec", enum."prec"="%_4p"}, enum."τ11"={enum."name"="τ11", enum."nameL"="tau11", enum."units"="sec", enum."prec"="%_4p"}, enum."τ12"={enum."name"="τ12", enum."nameL"="tau12", enum."units"="sec", enum."prec"="%_4p"}, enum."τ22"={enum."name"="τ22", enum."nameL"="tau22", enum."units"="sec", enum."prec"="%_4p"}, enum."τN1"={enum."name"="τN1", enum."nameL"="tauN1", enum."units"="sec", enum."prec"="%_4p"}, enum."τN2"={enum."name"="τN2", enum."nameL"="tauN2", enum."units"="sec", enum."prec"="%_4p"}, enum."σηlogτ1"={enum."name"="σηlogτ1", enum."nameL"="sigmaetalogtau1", enum."units"="au", enum."prec"="%_4p"}, enum."σηlogτS"={enum."name"="σηlogτS", enum."nameL"="sigmaetalogtauS", enum."units"="au", enum."prec"="%_4p"}, enum."σηlogτN"={enum."name"="σηlogτN", enum."nameL"="sigmaetalogtauN", enum."units"="au", enum."prec"="%_4p"}, enum."σlogτ1"={enum."name"="σlogτ1", enum."nameL"="sigmalogtau1", enum."units"="au", enum."prec"="%_4p"}, enum."σlogτS"={enum."name"="σlogτS", enum."nameL"="sigmalogtauS", enum."units"="au", enum."prec"="%_4p"}, enum."σlogτN"={enum."name"="σlogτN", enum."nameL"="sigmalogtauN", enum."units"="au", enum."prec"="%_4p"}, enum."σητ1"={enum."name"="σητ1", enum."nameL"="sigmaetatau1", enum."units"="sec", enum."prec"="%_4p"}, enum."σητS"={enum."name"="σητS", enum."nameL"="sigmaetatauS", enum."units"="sec", enum."prec"="%_4p"}, enum."σητN"={enum."name"="σητN", enum."nameL"="sigmaetatauN", enum."units"="sec", enum."prec"="%_4p"}, enum."noiseT"={enum."name"="noiseT", enum."nameL"="noiseT", enum."units"="au", enum."prec"="%_4p"}, enum."plain"={enum."name"="plain", enum."nameL"="plain", enum."units"="au", enum."prec"="%_4p"}, enum."vproj"={enum."name"="vproj", enum."nameL"="vproj", enum."units"="V", enum."prec"="%_4p"}}
  out "constrained \nfilename lookup":map{i32, string}(c390)={0="008_040924", 1="003_041124", 2="004_042224", 3="005_042224", 4="006_042224", 5="007_042224", 6="010_040924", 7="008_042224", 8="013_041024", 9="004_041124", 10="009_042224", 11="006_041124", 12="011_040924", 13="010_042224", 14="005_041124", 15="012_041024", 16="011_041024", 17="002_041024", 18="010_041024", 19="009_041024", 20="007_041124", 21="003_041024", 22="008_041124", 23="008_041024", 24="007_041024", 25="010_041124", 26="003_041224", 27="004_041224", 28="005_041224", 29="006_041224", 30="007_041224", 31="008_041224", 32="009_041224", 33="009_041124", 34="011_041124", 35="003_042424", 36="004_041024", 37="011_042224", 38="013_042224", 39="006_041024", 40="002_041224", 41="002_042424", 42="004_042424", 43="005_041024"}
  out "cursor x selector":map{T4, dbl}(c390)={enum."T (K)"=15.0, enum."B (T)"=60.0, enum."θ (deg)"=153.0}
  # "Basic NHMFL TDO routine\nv. 0.5       F. F. Balakirev\n\nmessed with by Arkady!"
  # "Background file is either an ASCII *.dat file produced by TDO earlier\nor *.fit file containing single column of polynomial fit coeficients.\n1st row in fit file is a text header, which is ingnored. Result is saved in a \n\"*diff.dat\" file in the output folder\nExample \"PDO1.fit\": \n\nFit y=A_i*x^i, starting with A_0\n3.25637E7\n2132.56863\n-12.60591\n-2.01013\n-0.04452\n-3.23119E-4"
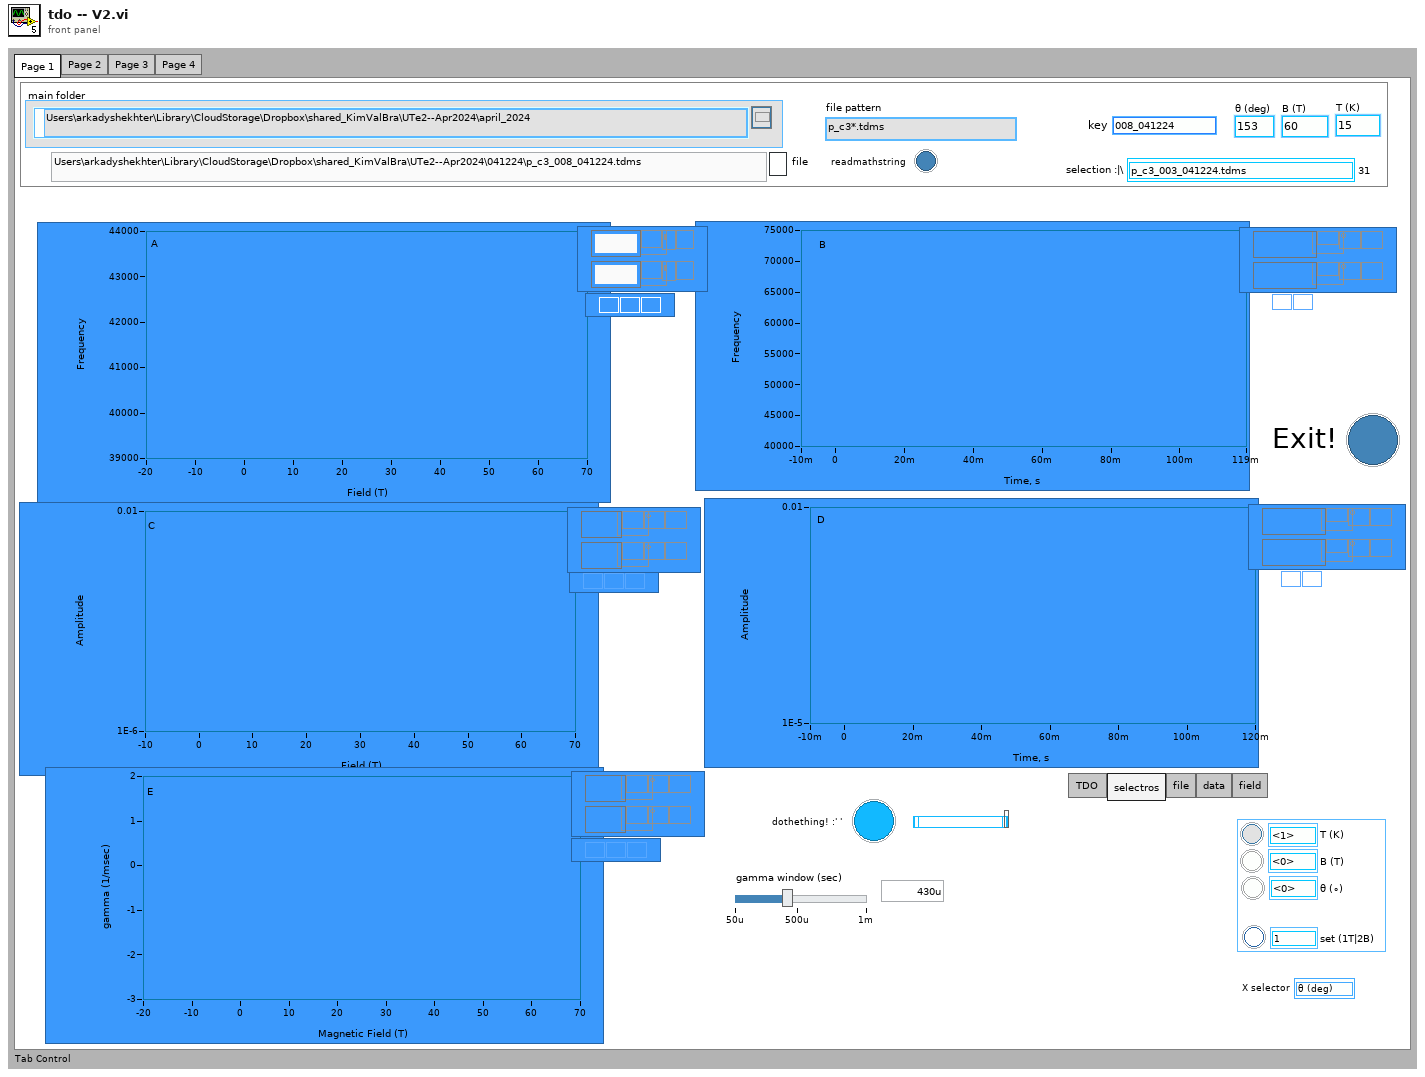
[diagram p1: front panel]
types:
  T1 = enum32{"TDO ", "selectros", "file", "data", "field"}
  T2 = enum16{"Power spectrum", "Tone detection", "Peak-to-peak fit"}
  T3 = cluster{"ignore set of !":bool, "set (1T|2B)":i32, "ignore θ !":bool, "ignore B !":bool, "T (K)":dbl, "ignore T !":bool, "θ (∘)":dbl, "B (T)":dbl, "lookup":cluster{"set of lookup":map{i32, dbl}, "all set of":set{dbl}, "T lookup":map{i32, dbl}, "θ lookup":map{i32, dbl}, "B lookup":map{i32, dbl}, "all T's":set{dbl}, "all θ's":set{dbl}, "all B's":set{dbl}, "all sides":set{dbl}, "side lookup":map{i32, dbl}}}
  T4 = typedef "3-lorentzian-parameters.ctl" = enum16{"ζ", "τ1", "τS", "τN", "τC", "κ0", "m1", "m2", "m3", "T (K)", "B (T)", "θ (deg)", "side (S|R)", "set of (B|T)", "Re(offset)", "Im(offset)", "στ1", "στ1-", "στ1+", "στS", "στS-", "στS+", "στN", "στN-", "στN+", "τ11", "τ12", "τ21", "τ22", "τN1", "τN2", "σηlogτ1", "σηlogτS", "σηlogτN", "σlogτ1", "σlogτS", "σlogτN", "σητ1", "σητS", "σητN", "noiseT", "plain", "vproj"}
  T5 = cluster{"Clip IIR filter ramps, in 1/Tc units":dbl, "Two-pass & flip":bool, "IIR filter specifications":cluster{"Topology":enum16{"Off", "Butterworth", "Chebyshev", "Inverse Chebyshev", "Elliptic", "Bessel"}, "Type":enum16{"Lowpass", "Highpass", "Bandpass", "Bandstop"}, "Order":i32, "Lower Fc":dbl, "Upper Fc":dbl, "PB Ripple":dbl, "SB Attenuation":dbl}}
  T6 = typedef "filename-action.ctl" = enum16{"rewrite", "parse", "force pattern", "uniquenum", "get T", "get B", "get ind", "get deg", "get name", "get folder", "get extension", "get basename", "get side", "get setof", "getID", "getIDStock", "remove prefix", "get36thing", "getplain", "getvproj"}
  T7 = typedef "nameformattingitem.ctl" = enum16{"name", "nameL", "units", "prec"}
  T8 = typedef "eventvkey.ctl" = enum16{"ASCII", "Enter", "Return", "Shift", "Ctrl", "Alt", "Cmd", "Opt", "Caps", "NumLock", "Clear", "Break", "Up", "Down", "Left", "Right", "Insert", "Delete", "Home", "End", "PageUp", "PageDown", "Escape", "Help", "Pause", "ScrollLock", "F1", "F2", "F3", "F4", "F5", "F6", "F7", "F8", "F9", "F10", "F11", "F12", "F13", "F14", "F15", "F16", "F17", "F18", "F19", "F20", "F21", "F22", "F23", "F24", "Play", "VolumeUp", "VolumeDown", "Mute", "Two Byte Char"}
  T9 = enum16{"Off", "Butterworth", "Chebyshev", "Inverse Chebyshev", "Elliptic", "Bessel"}
  T10 = typedef "Data window.ctl" = cluster{"Start":i64, "Length":i64, "Channel numbers":i64[], "Channel name":string, "Group name":string}
  T11 = typedef "interpolation state - real.ctl" = cluster{"Array ":dbl[], "actual size":i32, "requested size":i32}
  T12 = typedef "agregator -- action.ctl" = enum16{"append", "interpolate", "empty!", "force", "init", "scale", "read last"}
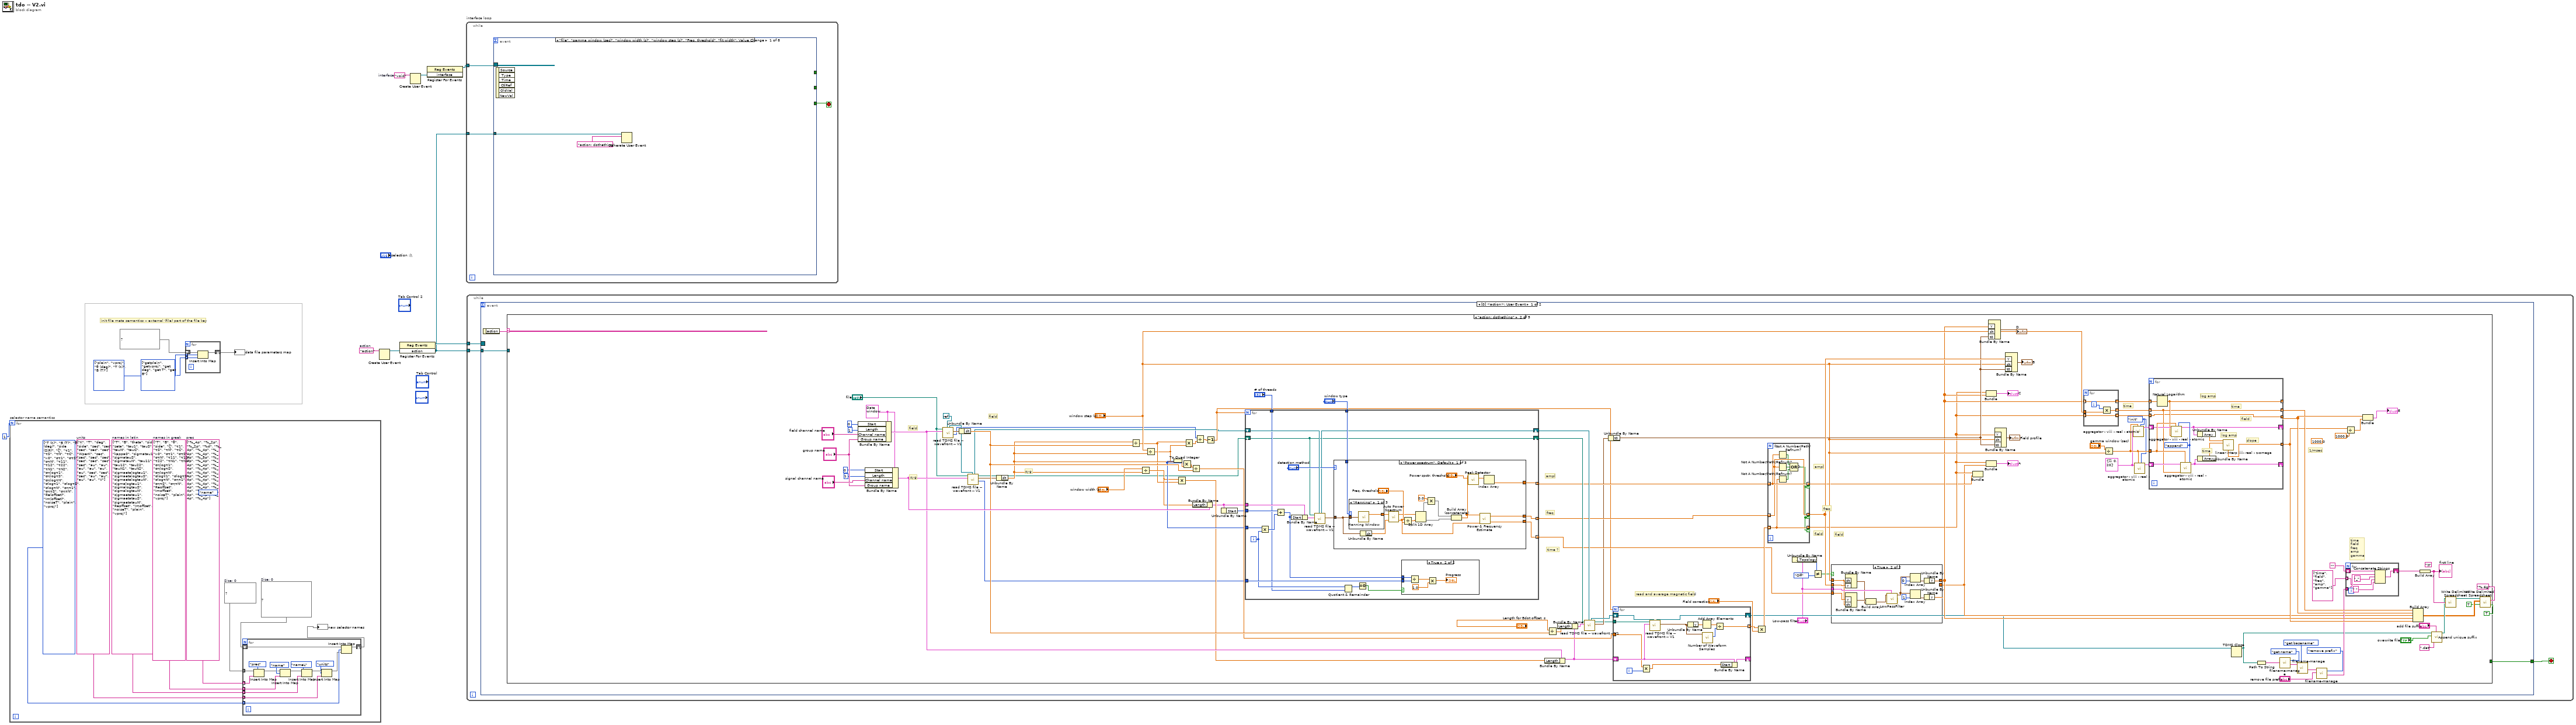
[diagram p0: block diagram]
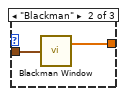
[diagram p5: hidden frame]
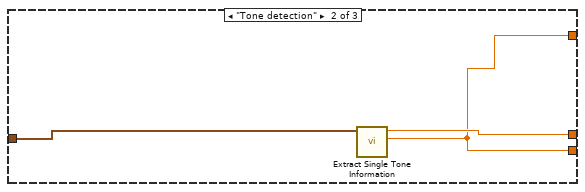
[diagram p7: hidden frame]
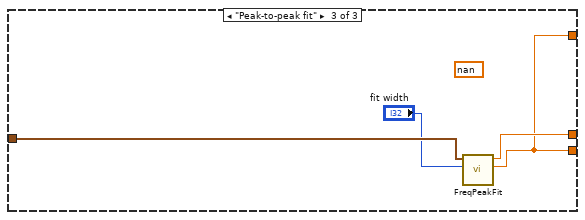
[diagram p8: hidden frame]
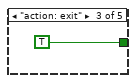
[diagram p9: hidden frame]
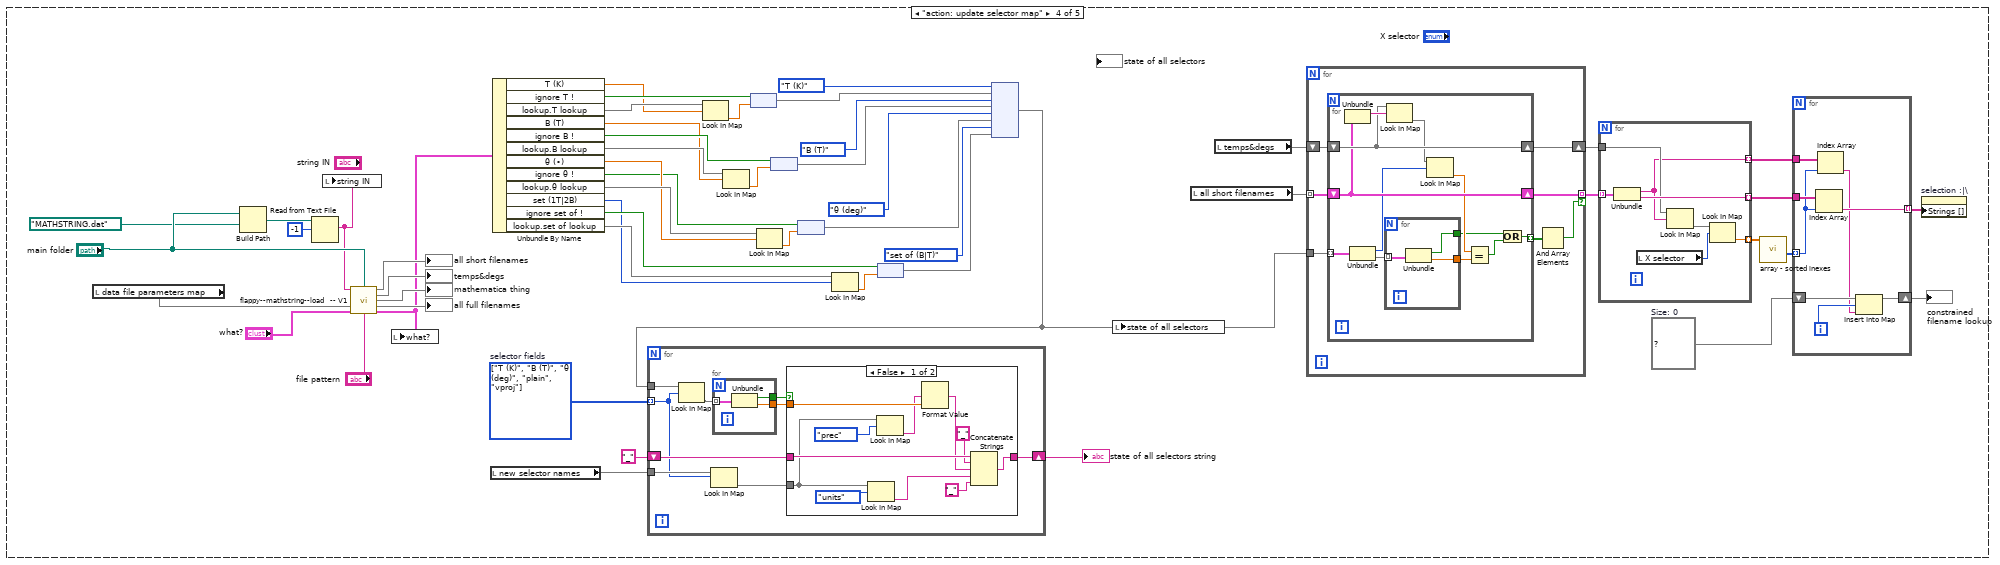
[diagram p10: hidden frame]
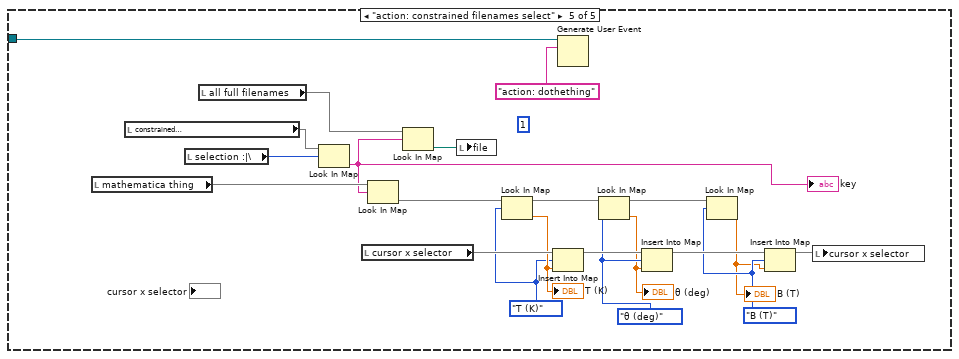
[diagram p12: hidden frame]
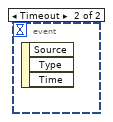
[diagram p13: hidden frame]
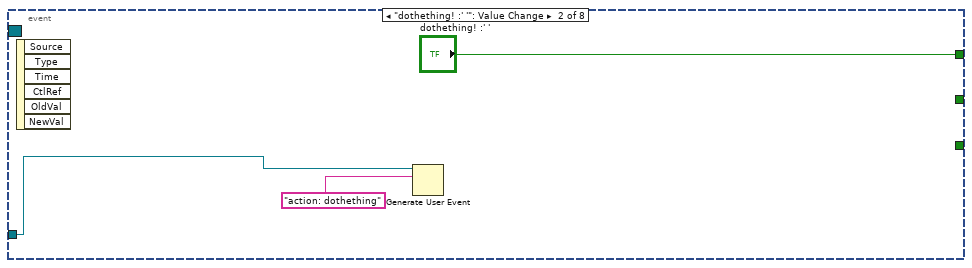
[diagram p14: hidden frame]
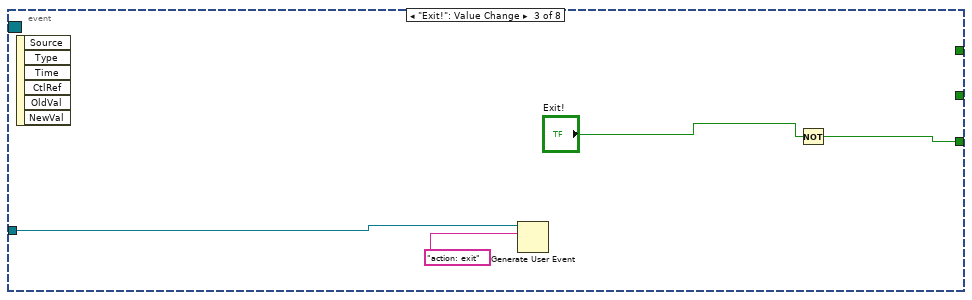
[diagram p15: hidden frame]
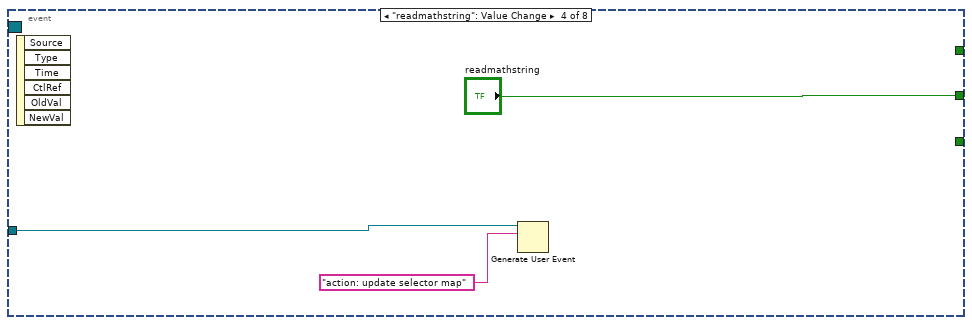
[diagram p16: hidden frame]
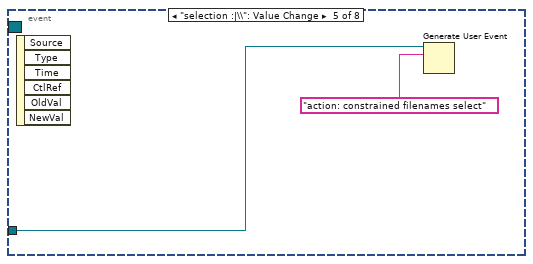
[diagram p17: hidden frame]
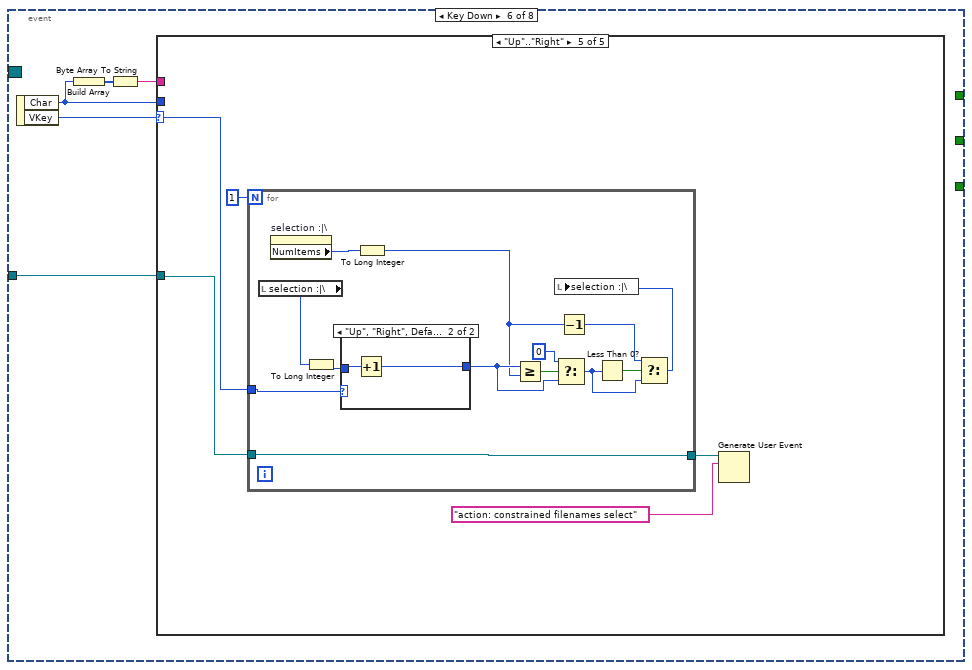
[diagram p18: hidden frame]
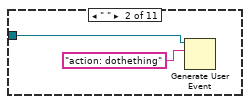
[diagram p20: hidden frame]
diagram:
  w5 = T6[] [enum."getplain", enum."getvproj", enum."get deg", enum."get T", enum."get B"] items=["rewrite", "parse", "force pattern", "uniquenum", "get T", "get B", "get ind", "get deg", "get name", "get folder", "get extension", "get basename", "get side", "get setof", "getID", "getIDStock", "remove prefix", "get36thing", "getplain", "getvproj"]
  w6 = T4[] [enum."plain", enum."vproj", enum."θ (deg)", enum."T (K)", enum."B (T)"] items=["ζ", "τ1", "τS", "τN", "τC", "κ0", "m1", "m2", "m3", "T (K)", "B (T)", "θ (deg)", "side (S|R)", "set of (B|T)", "Re(offset)", "Im(offset)", "στ1", "στ1-", "στ1+", "στS", "στS-", "στS+", "στN", "στN-", "στN+", "τ11", "τ12", "τ21", "τ22", "τN1", "τN2", "σηlogτ1", "σηlogτS", "σηlogτN", "σlogτ1", "σlogτS", "σlogτN", "σητ1", "σητS", "σητN", "noiseT", "plain", "vproj"]
  w9 = "void"  # interface
  w11 = "action"  # action
  # "init file meta semantics -- external (file) part of the file key"
  n1 = for "selector name semantics" {
    N: 1 -> [_]
    w13 = string[] ["%_4p", "%_2p", "%_2p", "%d", "%_4p", "%_4p", "%_4p", "%_4p", "%_4p", "%_5p", "%_4p", "%_4p", "%_4p", "%_4p", "%_4p", "%_4p", "%_4p", "%_4p", "%_4p", "%_4p", "%_4p", "%_4p", "%_4p", "%_4p", "%_4p", "%_4p", "%_4p", "%_4p", "%_4p", "%_4p", "%_4p", "%_4p"]  # prec
    w16 = map{T7, string} {}  # Size: 0
    (unwired) nameformattingitem."name" ("name formatting item")
    w14 = string[] ["K", "T", "deg", "side", "sec", "sec", "sec", "sec", "sec", "WperK", "sec", "sec", "sec", "sec", "sec", "sec", "sec", "sec", "au", "au", "au", "au", "au", "au", "sec", "sec", "sec", "au", "au", "au", "au", "V"]  # units
    w17 = string[] ["T", "B", "theta", "side", "zeta", "tau1", "tauS", "tauN", "tauC", "kappa0", "sigmatau1", "sigmatauS", "sigmatauN", "tau11", "tau12", "tau22", "tauN1", "tauN2", "sigmaetalogtau1", "sigmaetalogtauS", "sigmaetalogtauN", "sigmalogtau1", "sigmalogtauS", "sigmalogtauN", "sigmaetatau1", "sigmaetatauS", "sigmaetatauN", "Reoffset", "Imoffset", "noiseT", "plain", "vproj"]  # names in latin
    w15 = string[] ["T", "B", "θ", "side", "ζ", "τ1", "τS", "τN", "τC", "κ0", "στ1", "στS", "στN", "τ11", "τ12", "τ22", "τN1", "τN2", "σηlogτ1", "σηlogτS", "σηlogτN", "σlogτ1", "σlogτS", "σlogτN", "σητ1", "σητS", "σητN", "Reoffset", "Imoffset", "noiseT", "plain", "vproj"]  # names in greek
    w19 = map{T4, map{T7, string}} {}  # Size: 0
    w18 = T4[] [enum."T (K)", enum."B (T)", enum."θ (deg)", enum."side (S|R)", enum."ζ", enum."τ1", enum."τS", enum."τN", enum."τC", enum."κ0", enum."στ1", enum."στS", enum."στN", enum."τ11", enum."τ12", enum."τ22", enum."τN1", enum."τN2", enum."σηlogτ1", enum."σηlogτS", enum."σηlogτN", enum."σlogτ1", enum."σlogτS", enum."σlogτN", enum."σητ1", enum."σητS", enum."σητN", enum."Re(offset)", enum."Im(offset)", enum."noiseT", enum."plain", enum."vproj"] items=["ζ", "τ1", "τS", "τN", "τC", "κ0", "m1", "m2", "m3", "T (K)", "B (T)", "θ (deg)", "side (S|R)", "set of (B|T)", "Re(offset)", "Im(offset)", "στ1", "στ1-", "στ1+", "στS", "στS-", "στS+", "στN", "στN-", "στN+", "τ11", "τ12", "τ21", "τ22", "τN1", "τN2", "σηlogτ1", "σηlogτS", "σηlogτN", "σlogτ1", "σlogτS", "σlogτN", "σητ1", "σητS", "σητN", "noiseT", "plain", "vproj"]
    n2 = for {
      shift-right: [w34] -> w12
      shift-left: w19 -> [w35]
      tunnel: w17 -> [w25] mode=indexing
      tunnel: w18 -> [w33] mode=indexing
      tunnel: w16 -> [w23]
      tunnel: w15 -> [w24] mode=indexing
      tunnel: w14 -> [w26] mode=indexing
      tunnel: w13 -> [w22] mode=indexing
      n3 = Insert Into Map(map in=w23, key=nameformattingitem."prec", value=w22) -> (map out=w21:map{T7, string})  [unwired: 2 out]
      n4 = Insert Into Map(map in=w21, key=nameformattingitem."name", value=w24) -> (map out=w32:map{T7, string})  [unwired: 2 out]
      n5 = Insert Into Map(map in=w32, key=nameformattingitem."nameL" ("name formatting item"), value=w25) -> (map out=w31:map{T7, string})  [unwired: 2 out]
      n6 = Insert Into Map(map in=w31, key=nameformattingitem."units" ("name formatting item"), value=w26) -> (map out=w30:map{T7, string})  [unwired: 2 out]
      n7 = Insert Into Map(map in=w35, key=w33, value=w30) -> (map out=w34:map{T4, map{T7, string}})  [unwired: 2 out]
    }
    "new selector names" <- w12
  }
  n8 = for {
    shift-right: [w38] -> w3
    shift-left: map{T4, T6} {} ("data file parameters map") -> [w39]
    tunnel: w6 -> [w37] mode=indexing
    tunnel: w5 -> [w36] mode=indexing
    n9 = Insert Into Map(map in=w39, key=w37, value=w36) -> (map out=w38:map{T4, T6})  [unwired: 2 out]
  }
  "data file parameters map" <- w3
  n10 = Create User Event(user event datatype=w11) -> (user event=w1:refnum<user-event>)  [unwired: 1 in, 1 out]
  n11 = register-events(w1) -> (reference out=w7:refnum<event-registration>)  [unwired: 2 in, 1 out]
  n12 = Create User Event(user event datatype=w9) -> (user event=w8:refnum<user-event>)  [unwired: 1 in, 1 out]
  n13 = register-events(w8) -> (reference out=w10:refnum<event-registration>)  [unwired: 2 in, 1 out]
  n14 = while "interface loop" {
    tunnel: w10 -> [w42]
    tunnel: w1 -> [w40]
    stop <- w41 stop-if-true
    n15 = event shown="[0] \"file\", \"gamma window (sec)\", \"window width (s)\", \"window step (s)\", \"Freq. threshold\", \"fit width\": Value Change" {
      selector: w42 -> [_ _ _ _ _ _ _ _]
      dyn-events: _ -> [_ _ _ _ _ _ _ _]
      timeout: _ -> [_ _ _ _ _ _ _ _]
      tunnel: [_ _ w48 _ _ _ _ w88] -> w41
      tunnel: w40 -> [w44 w45 w50 w54 w55 w57 _ _]
      tunnel: [_ "dothething! :' '" _ _ _ _ _ _] -> _
      tunnel: [_ _ _ "readmathstring" _ _ _ _] -> _
      event "file", "gamma window (sec)", "window width (s)", "window step (s)", "Freq. threshold", "fit width": Value Change {
        n16 = event-data() -> ()  [unwired: 1 in, 6 out]
        n17 = Generate User Event(user event=w44, event data cluster="action: dothething" ("event data")) -> ()  [unwired: 2 in, 2 out]
      }
      event "dothething! :' '": Value Change {
        n18 = event-data() -> ()  [unwired: 1 in, 6 out]
        n19 = Generate User Event(user event=w45, event data cluster="action: dothething" ("event data")) -> ()  [unwired: 2 in, 2 out]
      }
      event "Exit!": Value Change {
        n20 = event-data() -> ()  [unwired: 1 in, 6 out]
        n21 = Generate User Event(user event=w50, event data cluster="action: exit" ("event data")) -> ()  [unwired: 2 in, 2 out]
        n22 = Not(x="Exit!") -> (.not. x?=w48:bool)
      }
      event "readmathstring": Value Change {
        n23 = event-data() -> ()  [unwired: 1 in, 6 out]
        n24 = Generate User Event(user event=w54, event data cluster="action: update selector map" ("event data")) -> ()  [unwired: 2 in, 2 out]
      }
      event "selection :|\\": Value Change {
        n25 = event-data() -> ()  [unwired: 1 in, 6 out]
        n26 = Generate User Event(user event=w55, event data cluster="action: constrained filenames select" ("event data")) -> ()  [unwired: 2 in, 2 out]
      }
      event Key Down {
        n27 = event-data() -> ("Char"=w59:i16, "VKey"=w61:T8)  [unwired: 1 in]
        n28 = Build Array(w59) -> (w60:i16[])
        n29 = Byte Array To String(unsigned byte array=w60) -> (string=w58:string)
        n30 = case shown="\"Up\"..\"Right\"" w61 {
          selector: w61 -> [_ _ _ _ w66]
          tunnel: w59 -> [_ _ _ _ _]
          tunnel: w58 -> [w63 _ _ _ _]
          tunnel: w57 -> [w62 _ _ _ w67]
          frame "ASCII", Default {
            n31 = case shown="\"0\", Default" w63 {
              tunnel: w62 -> [_ w64 _ _ _ _ _ _ _ _ _]
              frame "0", Default {
              }
              frame " " {
                n32 = Generate User Event(user event=w64, event data cluster="action: dothething" ("event data")) -> ()  [unwired: 2 in, 2 out]
              }
              frame "s" {
              }
              frame "l" {
              }
              frame "p" {
              }
              frame "?" {
              }
              frame "+", "-", "<", ">" {
              }
              frame "c" {
              }
              frame "t" {
              }
              frame "r" {
              }
              frame "d" {
              }
            }
          }
          frame "Escape" {
          }
          frame "PageUp" {
          }
          frame "PageDown" {
          }
          frame "Up".."Right" {
            n33 = for {
              N: 1 -> [_]
              tunnel: w66 -> [w83]
              tunnel: w67 -> [w82]
              tunnel: [w82] -> w68
              n34 = local read "selection :|\\"() -> (w75:u16)
              n35 = property on="selection :|\\" class="Ring (strict)"() -> ("NumItems"=w71:u32)  [unwired: 2 in, 2 out]
              n36 = To Long Integer(number=w75) -> (32bit integer=w74:i32)
              n37 = case shown="\"Up\", \"Right\", Default" w83 {
                tunnel: w74 -> [w85 w87]
                tunnel: [w84 w86] -> w79
                frame "Down", "Left" {
                  n38 = Decrement(x=w85) -> (x-1=w84:i32)
                }
                frame "Up", "Right", Default {
                  n39 = Increment(x=w87) -> (x+1=w86:i32)
                }
              }
              n40 = To Long Integer(number=w71) -> (32bit integer=w73:i32)
              n41 = Greater Or Equal?(x=w79, y=w73) -> (x >= y?=w81:bool)
              n42 = Select(t=u16 0 ("lower limit"), s=w81, f=w79) -> (s? t:f=w76:i32)
              n43 = Decrement(x=w73) -> (x-1=w77:i32)
              n44 = Less Than 0?(x=w76) -> (x < 0?=w78:bool)
              n45 = Select(t=w77, s=w78, f=w76) -> (s? t:f=w72:i32)
              n46 = local write "selection :|\\"(w72) -> ()
            }
            n47 = Generate User Event ("action User Event")(user event=w68, event data cluster="action: constrained filenames select" ("event data")) -> ()  [unwired: 2 in, 2 out]
          }
        }
      }
      event Timeout {
        n48 = event-data() -> ()  [unwired: 1 in, 3 out]
      }
      event User Event {
        n49 = event-data() -> ("interface"=w89:string)  [unwired: 1 in]
        n50 = case shown="\"False\", Default" w89 {
          tunnel: [_ TRUE] -> w88
          frame "False", Default {
          }
          frame "interface: exit" {
          }
        }
      }
    }
  }
  n51 = while {
    tunnel: w7 -> [w93]
    tunnel: w1 -> [w91]
    stop <- w92 stop-if-true
    n52 = event shown="[0] <action>: User Event" {
      selector: w93 -> [_ _]
      dyn-events: _ -> [_ _]
      timeout: _ -> [_ _]
      tunnel: [w95 _] -> w92
      tunnel: w91 -> [w94 _]
      event User Event {
        n53 = event-data() -> ("action"=w96:string)  [unwired: 1 in]
        n54 = case shown="\"action: dothething\"" w96 {
          tunnel: [_ _ TRUE _ _] -> w95
          tunnel: w94 -> [_ _ _ _ w443]
          frame "False", Default {
          }
          frame "action: dothething" {
            w115 = T10 {"Start"=0, "Length"=500000, "Channel numbers"=[0], "Channel name"="", "Group name"="Untitled"} ("Data window")
            (unwired) 1000.0
            (unwired) "\t"
            w99 = T11 {"Array "=[], "actual size"=0, "requested size"=20} ("state IN")
            w100 = agregator_--_action."init" ("aggregator action")
            # "syg"
            # "field"
            # "syg"
            # "field"
            # "time"
            # "a"
            # "time ?"
            # "read and average magnetic field"
            # "field"
            # "freq"
            # "freq"
            # "ampl"
            # "field"
            # "ampl"
            # "1/msec"
            # "time \nfield\nfreq\namp\ngamma"
            n55 = Bundle By Name(cluster=w115, "Start"=i64 0, "Length"=i64 1, "Channel name"="field channel name", "Group name"="group name") -> (w200:T10)
            n56 = Bundle By Name(cluster=w115, "Start"=i64 0, "Length"=i64 1, "Channel name"="signal channel name", "Group name"="group name") -> (w201:T10)
            n57 = call "read TDMS file -- wavefront -- V1.vi"("tdms file in"=refnum<k0> refnum, "Data window"=w200, "Input file path"="file") -> ("1st channel length"=w117:u64, "Data out"=w122:waveform(dbl), "tdms file out"=w120:refnum<k34>)  [unwired: 5 in, 1 out]
            n58 = Unbundle By Name(w122) -> ("dt"=w172:dbl)
            n59 = call "read TDMS file -- wavefront -- V1.vi"("tdms file in"=w120, "Data window"=w201, "Input file path"="file") -> ("1st channel length"=w118:u64, "Data out"=w123:waveform(dbl), "Actual input file path"=w116:path, "tdms file out"=w119:refnum<k34>)  [unwired: 5 in]
            n60 = Unbundle By Name(w123) -> ("dt"=w171:dbl)
            n61 = Divide(x=w171, y=w172) -> (x/y=w145:dbl)
            n62 = Divide(x="window width (s)", y=w171) -> (x/y=w150:dbl)
            n63 = Divide(x="window step (s)", y=w171) -> (x/y=w129:dbl)
            n64 = To Quad Integer(1:w129) -> (0:w151:i64)
            n65 = Multiply(x=w150, y=w145) -> (x*y=w149:dbl)
            n66 = Multiply(x=w151, y=w171) -> (x*y=w152:dbl)
            n67 = Multiply(x=w145, y=w129) -> (x*y=w138:dbl)
            n68 = Divide(x=w152, y=w172) -> (x/y=w153:dbl)
            n69 = Bundle By Name(cluster=w201, "Length"=w150) -> (w146:T10)
            n70 = Divide(x=w117, y=w138) -> (x/y=w124:dbl)
            n71 = Decrement(x=w124) -> (x-1=w140:dbl)
            n72 = Unbundle By Name(w146) -> ("Start"=w147:i64)
            n73 = for {
              N: w140 -> [_]
              tunnel: [w279] -> w156 mode=indexing
              tunnel: [w281] -> w155 mode=indexing
              tunnel: [w280] -> w157 mode=indexing
              tunnel: w151 -> [w276]
              tunnel: w118 -> [w278]
              tunnel: w146 -> [w275]
              tunnel: w147 -> [w274]
              tunnel: "window type" -> [w272]
              tunnel: "# of threads" -> [w265]
              shift-right: [w263] -> w194
              shift-left: w119 -> [w266]
              shift-right: [w262] -> w193
              shift-left: w116 -> [w262]
              i -> [w269]
              n74 = Multiply(x=w276, y=w269) -> (x*y=w270:i64)
              n75 = Add(x=w274, y=w270) -> (x+y=w271:i64)
              n76 = Bundle By Name(cluster=w275, "Start"=w271) -> (w273:T10)
              n77 = call "read TDMS file -- wavefront -- V1.vi"("tdms file in"=w266, "Data window"=w273, "Input file path"=w262) -> ("Data out"=w277:waveform(dbl), "tdms file out"=w263:refnum<k34>)  [unwired: 5 in, 2 out]
              n78 = case shown="\"Power spectrum\", Default" "detection method" {
                tunnel: [w303 w310 w313] -> w281
                tunnel: [w290 w310 w313] -> w280
                tunnel: w277 -> [w302 w311 w316]
                tunnel: [w292 w312 w315] -> w279
                tunnel: w272 -> [w293 _ _]
                frame "Power spectrum", Default {
                  n79 = case shown="\"Hanning\"" w293 {
                    tunnel: [w306 w308 w309] -> w304
                    tunnel: w302 -> [w305 w307 w309]
                    frame "Hanning" {
                      n80 = call-poly <vilib>:"Hanning Window.vi"("X"=w305) -> ("Windowed X"=w306:dbl[])  [unwired: 1 out]
                    }
                    frame "Blackman" {
                      n81 = call-poly <vilib>:"Blackman Window.vi"("X"=w307) -> ("Windowed X"=w308:dbl[])  [unwired: 1 out]
                    }
                    frame "Box" {
                    }
                  }
                  n82 = Unbundle By Name(w302) -> ("dt"=w301:dbl)
                  n83 = call <vilib>:"Auto Power Spectrum.vi"("dt"=w301, "Signal (V)"=w304) -> ("df"=w291:dbl, "Power Spectrum (V^2 rms)"=w299:dbl[])
                  n84 = Divide(x="Freq. threshold", y=w291) -> (x/y=w298:dbl)
                  n85 = Split 1D Array(array=w299, index=w298) -> (first subarray=w295:dbl[], second subarray=w297:dbl[])
                  n86 = Multiply(x=0.0 ("element"), y=w295) -> (x*y=w294:dbl[])
                  n87 = Build Array (concatenate)(w294, w297) -> (w289:dbl[])
                  n88 = call <vilib>:"Peak Detector.vi"("threshold"="Power spctr. threshold", "X"=w289) -> ("Amplitudes"=w287:dbl[])  [unwired: 5 in, 4 out]
                  n89 = call <vilib>:"Power & Frequency Estimate.vi"("df"=w291, "Power Spectrum (V^2 rms)"=w289) -> ("est power peak"=w303:dbl, "est frequency peak"=w292:dbl)  [unwired: 3 in, 1 out]
                  n90 = Index Array(array=w287) -> (element=w290:dbl)  [unwired: 1 in]
                }
                frame "Tone detection" {
                  n91 = call-poly <vilib>:"Extract Single Tone Information.vi"("time signal in"=w311) -> ("detected amplitude"=w310:dbl, "detected frequency"=w312:dbl)  [unwired: 3 in, 6 out]
                }
                frame "Peak-to-peak fit" {
                  (unwired) nan
                  n92 = call "FreqPeakFit.vi"("Peak fit width"="fit width", "Waveform"=w316) -> ("Amplitude"=w313:dbl, "PeakFreqOut"=w315:dbl)  [unwired: 1 in, 5 out]
                }
              }
              n93 = Quotient & Remainder(x=w269, y=w265) -> (x-y*floor(x/y)=w268:i32)  [unwired: 1 out]
              n94 = Equal To 0?(x=w268) -> (x = 0?=w267:bool)
              n95 = case shown="True" w267 {
                tunnel: w278 -> [_ w286]
                tunnel: w271 -> [_ w283]
                frame False {
                }
                frame True {
                  n96 = Divide(x=w283, y=w286) -> (x/y=w285:dbl)
                  n97 = Multiply(x=w285, y=1.0) -> (x*y=→"Progress":dbl)
                }
              }
            }
            n98 = Bundle By Name(cluster=w200, "Length"=w149) -> (w137:T10)
            n99 = Divide(x="Length for Bdot offset, s", y=w172) -> (x/y=w136:dbl)
            n100 = Bundle By Name(cluster=w137, "Length"=w136) -> (w141:T10)
            n101 = call "read TDMS file -- wavefront -- V1.vi"("tdms file in"=w194, "Data window"=w141, "Input file path"=w193) -> ("Data out"=w142:waveform(dbl), "Actual input file path"=w139:path, "tdms file out"=w143:refnum<k34>)  [unwired: 5 in, 1 out]
            n102 = Unbundle By Name(w142) -> ("t0"=w188:timestamp)
            n103 = for {
              N: w140 -> [_]
              shift-right: [w245] -> _
              shift-left: w137 -> [w244]
              tunnel: w153 -> [w237]
              tunnel: [w243] -> w160 mode=indexing
              tunnel: w139 -> [w242]
              shift-right: [w239] -> w144
              shift-left: w143 -> [w240]
              i -> [w238]
              n104 = Multiply(x=w237, y=w238) -> (x*y=w236:dbl)
              n105 = call "read TDMS file -- wavefront -- V1.vi"("tdms file in"=w240, "Data window"=w244, "Input file path"=w242) -> ("Data out"=w241:waveform(dbl), "tdms file out"=w239:refnum<k34>)  [unwired: 5 in, 2 out]
              n106 = Unbundle By Name(w241) -> ("Y"=w235:dbl[])
              n107 = Add Array Elements(numeric array=w235) -> (sum=w233:dbl)
              n108 = call-poly <vilib>:"Number of Waveform Samples.vi"("waveform in"=w241) -> ("number of samples"=w234:i32)  [unwired: 1 in, 9 out]
              n109 = Divide(x=w233, y=w234) -> (x/y=w243:dbl)
              n110 = Bundle By Name(cluster=w244, "Start"=w236) -> (w245:T10)
            }
            n111 = Multiply(x=w160, y="Field correction") -> (x*y=w162:dbl[])
            n112 = for {
              tunnel: w156 -> [w231] mode=indexing
              tunnel: w162 -> [w230] mode=indexing
              tunnel: w157 -> [w232] mode=indexing
              tunnel: [w232] -> w159 mode=indexing if=w226
              tunnel: [w231] -> w196 mode=indexing if=w226
              tunnel: [w230] -> w164 mode=indexing if=w226
              n113 = Not A Number/Path/Refnum?(number/path/refnum=w232) -> (NaN/Path/Refnum?=w229:bool)
              n114 = Not A Number/Path/Refnum?(number/path/refnum=w231) -> (NaN/Path/Refnum?=w228:bool)
              n115 = Not A Number/Path/Refnum?(number/path/refnum=w230) -> (NaN/Path/Refnum?=w227:bool)
              n116 = Compound Arithmetic op=OR(w229, w228, w227) -> (invert w226:bool)
            }
            n117 = Unbundle By Name("Low-pass filter") -> ("IIR filter specifications.Topology"=w130:T9)
            n118 = Not Equal?(x=w130, y=T9."Off" ("IIR filter specifications.Topology")) -> (x != y?=w131:bool)
            n119 = case shown="True" w131 {
              tunnel: "Low-pass filter" -> [_ w261]
              tunnel: w155 -> [w247 w259]
              tunnel: w196 -> [w246 w260]
              tunnel: "window step (s)" -> [_ w248]
              tunnel: [w246 w250] -> w158
              tunnel: [w247 w249] -> w186
              frame False {
              }
              frame True {
                n120 = Bundle By Name("dt"=w248, "Y"=w260) -> (w257:waveform(dbl))  [unwired: 1 out]
                n121 = Bundle By Name("Y"=w259, "dt"=w248) -> (w258:waveform(dbl))  [unwired: 1 out]
                n122 = Build Array(w258, w257) -> (w256:waveform(dbl)[])
                n123 = call "LowPassFilter.vi"("Low-pass filter"=w261, "signal(s) in"=w256) -> ("signal(s) out"=w255:waveform(dbl)[])  [unwired: 3 in, 6 out]
                n124 = Index Array(array=w255, index=0) -> (element=w252:waveform(dbl))
                n125 = Index Array(array=w255, index=1) -> (element=w251:waveform(dbl))
                n126 = Unbundle By Name(w252) -> ("Y"=w249:dbl[])
                n127 = Unbundle By Name(w251) -> ("Y"=w250:dbl[])
              }
            }
            n128 = Bundle(w164, w159) -> ()  [unwired: 2 out]
            n129 = Bundle(w164, "Y"=w186) -> (→"C":cluster{dbl[], "Y":dbl[]})  [unwired: 1 out]
            n130 = Bundle(w164, "Y"=w158) -> (→"A":cluster{dbl[], "Y":dbl[]})  [unwired: 1 out]
            n131 = Bundle By Name("Y"=w186, "dt"="window step (s)", "t0"=w188) -> (→"D":waveform(dbl))  [unwired: 1 out]
            n132 = Bundle By Name("Y"=w164, "dt"="window step (s)", "t0"=w188) -> (→"Field profile":waveform(dbl))  [unwired: 1 out]
            n133 = Bundle By Name("Y"=w196, "dt"="window step (s)", "t0"=w188) -> (→"B":waveform(dbl))  [unwired: 1 out]
            n134 = for {
              tunnel: w186 -> [w223] mode=indexing
              tunnel: "window step (s)" -> [w225]
              tunnel: [w224] -> w173 mode=indexing
              tunnel: [w223] -> w166 mode=indexing
              tunnel: [w222] -> w169 mode=indexing
              tunnel: w164 -> [w222] mode=indexing
              i -> [w221]
              n135 = Multiply(x=w221, y=w225) -> (x*y=w224:dbl)
            }
            n136 = Divide(x="gamma window (sec)", y="window step (s)") -> (x/y=w167:dbl)
            n137 = call "aggregator - viii - real - atomic.vi"("aggregator action"=w100, "requested size"=w167, "state IN"=w99) -> ("state OUT"=w168:T11)  [unwired: 5 in, 3 out]
            n138 = call "aggregator - viii - real - atomic.vi"("aggregator action"=w100, "requested size"=w167, "state IN"=w99) -> ("state OUT"=w165:T11)  [unwired: 5 in, 3 out]
            n139 = for {
              shift-right: [w214] -> _
              shift-left: w165 -> [w220]
              tunnel: w167 -> [w217]
              tunnel: w166 -> [w219] mode=indexing
              tunnel: w173 -> [w209] mode=indexing
              shift-right: [w215] -> _
              shift-left: w168 -> [w216]
              tunnel: [w211] -> w184 mode=indexing
              tunnel: [w210] -> _ mode=indexing
              tunnel: [w209] -> w191 mode=indexing
              tunnel: w169 -> [w208] mode=indexing
              tunnel: [w208] -> w192 mode=indexing
              w218 = agregator_--_action."append" ("aggregator action")
              # "field"
              # "slope"
              # "time"
              # "log amp"
              # "log amp"
              # "time"
              n140 = Natural Logarithm(1:w219) -> (0:w210:dbl)
              n141 = call "aggregator - viii - real - atomic.vi"("aggregator action"=w218, "requested size"=w217, "number"=w210, "state IN"=w216) -> ("state OUT"=w215:T11)  [unwired: 4 in, 3 out]
              n142 = call "aggregator - viii - real - atomic.vi"("aggregator action"=w218, "requested size"=w217, "number"=w209, "state IN"=w220) -> ("state OUT"=w214:T11)  [unwired: 4 in, 3 out]
              n143 = Unbundle By Name(w215) -> ("Array"=w212:dbl[])
              n144 = Unbundle By Name(w214) -> ("Array"=w213:dbl[])
              n145 = call "linear interp iiii- real - z-omega.vi"("z"=w212, "omega"=w213) -> ("slope"=w211:dbl)  [unwired: 4 in, 9 out]
            }
            n146 = TDMS Close(11:w144) -> (3:w177:path)  [unwired: 1 in, 1 out]
            n147 = Path To String(path=w177) -> (string=w178:string)
            n148 = call "filename-manage.vi"("filename-action"=filename-action."get name", "file name IN"=w178) -> ("string OUT"=w179:string)  [unwired: 7 in, 2 out]
            n149 = call "filename-manage.vi"("filename-action"=filename-action."get basename", "file name IN"=w179) -> ("string OUT"=w180:string)  [unwired: 7 in, 2 out]
            n150 = call "filename-manage.vi"("filename-action"=filename-action."remove prefix", "string IN"="remove file prefix", "file name IN"=w180) -> ("string OUT"=w182:string)  [unwired: 6 in, 2 out]
            n151 = Divide(x=w184, y=1000.0) -> (x/y=w185:dbl[])
            n152 = for {
              tunnel: string[] ["time", "field", "freq", "amp", "gamma"] -> [w203] mode=indexing
              shift-right: [w206] -> w183
              shift-left: "" ("format (%.3f)") -> [w207]
              tunnel: w182 -> [w205]
              n153 = Concatenate Strings(w207, w205, "_", w203, " ") -> (w206:string)
            }
            n154 = Bundle(w192, w185) -> (→"E":cluster{dbl[], dbl[]})  [unwired: 1 out]
            n155 = Build Array(w191, w192, w158, w186, w184) -> (w126:dbl[][])
            n156 = Build Array(w183) -> (w175:string[])
            "first line" <- w175
            n157 = call "Append unique suffix.vi"("Extention"=".dat", "Suffix"="add file suffix", "ovewrite ?"="ovewrite file?", "Path"=w177) -> ("Path out"=w174:path)  [unwired: 6 in, 1 out]
            n158 = call-poly <vilib>:"Write Delimited Spreadsheet.vi"("file path (dialog if empty)"=w174, "1D data"=w175) -> ("new file path (Not A Path if cancelled)"=w176:path)  [unwired: 12 in, 1 out]
            n159 = call-poly <vilib>:"Write Delimited Spreadsheet.vi"("file path (dialog if empty)"=w176, "format (%.3f)"="%.6g", "2D data"=w126, "append to file? (new file:F)"=TRUE, "transpose? (no:F)"=TRUE) -> ()  [unwired: 9 in, 2 out]
          }
          frame "action: exit" {
          }
          frame "action: update selector map" {
            w337 = map{i32, string} {}  # Size: 0
            w355 = T4[] [enum."T (K)", enum."B (T)", enum."θ (deg)", enum."plain", enum."vproj"] items=["ζ", "τ1", "τS", "τN", "τC", "κ0", "m1", "m2", "m3", "T (K)", "B (T)", "θ (deg)", "side (S|R)", "set of (B|T)", "Re(offset)", "Im(offset)", "στ1", "στ1-", "στ1+", "στS", "στS-", "στS+", "στN", "στN-", "στN+", "τ11", "τ12", "τ21", "τ22", "τN1", "τN2", "σηlogτ1", "σηlogτS", "σηlogτN", "σlogτ1", "σlogτS", "σlogτN", "σητ1", "σητS", "σητN", "noiseT", "plain", "vproj"]  # selector fields
            n160 = local read "data file parameters map"() -> (w319:map{T4, T6})
            n161 = Build Path(base path="main folder", name or relative path=path "MATHSTRING.dat") -> (appended path=w322:path)
            n162 = Read from Text File(file (use dialog)=w322, count=-1) -> (text=w323:string)  [unwired: 2 in, 3 out]
            n163 = local write "string IN"(w323) -> ()
            n164 = call "flappy--mathstring--load   -- V1.vi"("mathstring IN"=w323, "MAIN folder"="main folder", "data file parameters map"=w319, "what? IN"="what?", "data file pattern"="file pattern") -> ("all short filenames"=→"all short filenames":map{string, string}, "temps&degs"=→"temps&degs":map{string, map{T4, dbl}}, "mathematica thing"=→"mathematica thing":map{string, map{T4, dbl}}, "all full filenames"=→"all full filenames":map{string, path}, "what? OUT"=w318:T3)  [unwired: 6 in]
            n165 = local write "what?"(w318) -> ()
            n166 = local read "new selector names"() -> (w358:map{T4, map{T7, string}})
            n167 = Unbundle By Name(w318) -> ("T (K)"=w352:dbl, "ignore T !"=w354:bool, "lookup.T lookup"=w353:map{i32, dbl}, "B (T)"=w349:dbl, "ignore B !"=w351:bool, "lookup.B lookup"=w350:map{i32, dbl}, "θ (∘)"=w347:dbl, "ignore θ !"=w346:bool, "lookup.θ lookup"=w348:map{i32, dbl}, "set (1T|2B)"=w343:i32, "ignore set of !"=w344:bool, "lookup.set of lookup"=w345:map{i32, dbl})
            n168 = Look In Map(map=w353, key=w352) -> (value=w370:dbl)  [unwired: 1 in, 1 out]
            n169 = Look In Map(map=w350, key=w349) -> (value=w366:dbl)  [unwired: 1 in, 1 out]
            n170 = node(w354, w370) -> (w368:map{bool, dbl})
            n171 = Look In Map(map=w348, key=w347) -> (value=w364:dbl)  [unwired: 1 in, 1 out]
            n172 = node(w351, w366) -> (w365:map{bool, dbl})
            n173 = node(w346, w364) -> (w362:map{bool, dbl})
            n174 = Look In Map(map=w345, key=w343) -> (value=w361:dbl)  [unwired: 1 in, 1 out]
            n175 = node(w344, w361) -> (w359:map{bool, dbl})
            n176 = node(3-lorentzian-parameters."T (K)" ("Plost: sweep window"), w368, 3-lorentzian-parameters."B (T)" ("Plost: sweep window"), w365, 3-lorentzian-parameters."θ (deg)" ("Plost: sweep window"), w362, 3-lorentzian-parameters."set of (B|T)" ("Plost: sweep window"), w359) -> (w331:map{T4, map{bool, dbl}})
            n177 = for {
              tunnel: w358 -> [w409]
              shift-right: [w412] -> w356
              shift-left: "_" ("event data") -> [w411]
              tunnel: w355 -> [w408] mode=indexing
              tunnel: w331 -> [w406]
              n178 = Look In Map(map=w406, key=w408) -> (value=w414:map{bool, dbl})  [unwired: 1 in, 1 out]
              n179 = Look In Map(map=w409, key=w408) -> (value=w407:map{T7, string})  [unwired: 1 in, 1 out]
              n180 = for {
                tunnel: w414 -> [w429] mode=indexing
                tunnel: [w428] -> w413
                tunnel: [w427] -> w410
                n181 = Unbundle(w429) -> ("ignore T !"=w428:bool, "number OUT"=w427:dbl)
              }
              n182 = case shown="False" w413 {
                tunnel: [w425 w426] -> w412
                tunnel: w411 -> [w424 w426]
                tunnel: w410 -> [w421 _]
                tunnel: w407 -> [w417 _]
                frame False {
                  n183 = Look In Map(map=w417, key=nameformattingitem."units") -> (value=w418:string)  [unwired: 1 in, 1 out]
                  n184 = Look In Map(map=w417, key=nameformattingitem."prec") -> (value=w415:string)  [unwired: 1 in, 1 out]
                  n185 = Format Value(format string=w415, value (0)=w421) -> (output string=w420:string)  [unwired: 1 in]
                  n186 = Concatenate Strings(w424, "_" ("event data"), w420, w418, "_" ("event data")) -> (w425:string)
                }
                frame True {
                }
              }
            }
            "state of all selectors string" <- w356
            n187 = local write "state of all selectors"(w331) -> ()
            n188 = local read "all short filenames"() -> (w334:map{string, string})
            n189 = local read "temps&degs"() -> (w335:map{string, map{T4, dbl}})
            n190 = for {
              tunnel: w334 -> [w375] mode=indexing
              tunnel: [w375] -> w336 mode=indexing if=w371
              shift-right: [w374] -> w333
              shift-left: w335 -> [w374]
              tunnel: w331 -> [w372]
              n191 = for {
                tunnel: [w387] -> w373 mode=indexing
                shift-right: [w382] -> _
                shift-left: w375 -> [w382]
                shift-right: [w381] -> _
                shift-left: w374 -> [w381]
                tunnel: w372 -> [w380] mode=indexing
                n192 = Unbundle(w382) -> ("event data"=w386:string)  [unwired: 1 out]
                n193 = Unbundle(w380) -> ("Plost: sweep window"=w379:T4, "map"=w378:map{bool, dbl})
                n194 = for {
                  tunnel: w378 -> [w390] mode=indexing
                  tunnel: [w389] -> w376
                  tunnel: [w388] -> w377
                  n195 = Unbundle(w390) -> ("ignore T !"=w389:bool, "number OUT"=w388:dbl)
                }
                n196 = Look In Map(map=w381, key=w386) -> (value=w385:map{T4, dbl})  [unwired: 1 in, 1 out]
                n197 = Look In Map(map=w385, key=w379) -> (value=w384:dbl)  [unwired: 1 in, 1 out]
                n198 = Equal?(x=w384, y=w377) -> (x = y?=w383:bool)
                n199 = Or(x=w376, y=w383) -> (x .or. y?=w387:bool)
              }
              n200 = And Array Elements(Boolean array=w373) -> (logical AND=w371:bool)
            }
            n201 = for {
              tunnel: [w405] -> w340 mode=indexing
              tunnel: [w403] -> w338 mode=indexing
              tunnel: [w400] -> w342 mode=indexing
              tunnel: w336 -> [w402] mode=indexing
              tunnel: w333 -> [w401]
              n202 = Unbundle(w402) -> ("event data"=w400:string, "file pattern"=w405:string)
              n203 = local read "X selector"() -> (w399:T4)
              n204 = Look In Map(map=w401, key=w400) -> (value=w404:map{T4, dbl})  [unwired: 1 in, 1 out]
              n205 = Look In Map(map=w404, key=w399) -> (value=w403:dbl)  [unwired: 1 in, 1 out]
            }
            n206 = call "array - sorted inexes.vi"("x"=w338) -> ("index array"=w339:i32[])  [unwired: 9 in, 1 out]
            n207 = for {
              tunnel: w339 -> [w395] mode=indexing
              tunnel: w340 -> [w398]
              tunnel: [w397] -> w341 mode=indexing
              tunnel: w342 -> [w396]
              shift-right: [w391] -> w332
              shift-left: w337 -> [w394]
              i -> [w393]
              n208 = Index Array(array=w398, index=w395) -> (element=w397:string)
              n209 = Index Array(array=w396, index=w395) -> (element=w392:string)
              n210 = Insert Into Map(map in=w394, key=w393, value=w392) -> (map out=w391:map{i32, string})  [unwired: 2 out]
            }
            "constrained \nfilename lookup" <- w332
            n211 = property on="selection :|\\" class="Ring (strict)"("Strings []"=w341) -> ()  [unwired: 2 in, 2 out]
          }
          frame "action: constrained filenames select" {
            w432 = 3-lorentzian-parameters."B (T)" ("Plost: sweep window")
            w434 = 3-lorentzian-parameters."θ (deg)" ("Plost: sweep window")
            w435 = 3-lorentzian-parameters."T (K)" ("Plost: sweep window")
            (unwired) 1
            n212 = local read "mathematica thing"() -> (w438:map{string, map{T4, dbl}})
            n213 = local read "constrained \nfilename lookup"() -> (w445:map{i32, string})
            n214 = local read "selection :|\\"() -> (w446:u16)
            n215 = local read "all full filenames"() -> (w447:map{string, path})
            n216 = Look In Map(map=w445, key=w446) -> (value=w430:string)  [unwired: 1 in, 1 out]
            "key" <- w430
            n217 = local read "cursor x selector"() -> (w442:map{T4, dbl})
            n218 = Look In Map(map=w438, key=w430) -> (value=w437:map{T4, dbl})  [unwired: 1 in, 1 out]
            n219 = Look In Map(map=w447, key=w430) -> (value=w448:path)  [unwired: 1 in, 1 out]
            n220 = local write "file"(w448) -> ()
            n221 = Look In Map(map=w437, key=w435) -> (value=w436:dbl)  [unwired: 1 in, 1 out]
            "T (K)" <- w436
            n222 = Insert Into Map(map in=w442, key=w435, value=w436) -> (map out=w441:map{T4, dbl})  [unwired: 2 out]
            n223 = Generate User Event(user event=w443, event data cluster="action: dothething" ("event data")) -> ()  [unwired: 2 in, 2 out]
            n224 = Look In Map(map=w437, key=w434) -> (value=w433:dbl)  [unwired: 1 in, 1 out]
            "θ (deg)" <- w433
            n225 = Insert Into Map(map in=w441, key=w434, value=w433) -> (map out=w440:map{T4, dbl})  [unwired: 2 out]
            n226 = Look In Map(map=w437, key=w432) -> (value=w431:dbl)  [unwired: 1 in, 1 out]
            "B (T)" <- w431
            n227 = Insert Into Map(map in=w440, key=w432, value=w431) -> (map out=w439:map{T4, dbl})  [unwired: 2 out]
            n228 = local write "cursor x selector"(w439) -> ()
          }
        }
      }
      event Timeout {
        n229 = event-data() -> ()  [unwired: 1 in, 3 out]
      }
    }
  }
